vi "WriteConfiguration_Widget.vi"(7 "PythonConverter_GUI in":refnum<class "PythonConverter_GUI.lvclass">, 8 "error in":errorcluster, 11 "Control in":refnum<class "Control.lvclass">) -> (0 "error out":errorcluster, 3 "Control out":refnum<class "Control.lvclass">, 5 "PythonConverter_GUI out":refnum<class "PythonConverter_GUI.lvclass">)   [LabVIEW 2014, in "PythonConverter_GUI.lvclass"]
uses:
  PythonConverter_GUI.lvclass
  VI Interpreter/Classes/Control/Control.lvclass
  VI Interpreter/Classes/Control/Control.lvclass/Control.ctl
  PythonConverter_GUI.lvclass/PythonConverter_GUI.ctl
  PythonConfiguration/PythonConfiguration.lvclass/PythonConfiguration.ctl
  VI Interpreter/Classes/Boolean/Boolean.lvclass/Boolean.ctl
  VI Interpreter/Classes/Digital/Digital.lvclass/Digital.ctl
  VI Interpreter/Classes/Text/Text.lvclass/Text.ctl
  VI Interpreter/Classes/GraphChart/GraphChart.lvclass/GraphChart.ctl
  VI Interpreter/Classes/GraphScale/GraphScale.lvclass/GraphScale.ctl
  VI Interpreter/Classes/WaveformGraph/WaveformGraph.lvclass/WaveformGraph.ctl
  VI Interpreter/Classes/Knob/Knob.lvclass/Knob.ctl
  VI Interpreter/Classes/RotaryColorScale/RotaryColorScale.lvclass/RotaryColorScale.ctl
  VI Interpreter/Classes/NumericWithScale/NumericWithScale.lvclass/NumericWithScale.ctl
  VI Interpreter/Classes/Scale/Scale.lvclass/Scale.ctl
  VI Interpreter/Classes/String/String.lvclass/String.ctl
  VI Interpreter/Classes/IOName/IOName.lvclass/IOName.ctl
  VI Interpreter/Classes/Path/Path.lvclass/Path.ctl
  <vilib>/Utility/miscctls.llb/LVPositionTypeDef.ctl
  VI Interpreter/Classes/GObject/GObject.lvclass/GObject.ctl
  VI Interpreter/Classes/Combobox/Combobox.lvclass/Combobox.ctl
  VI Interpreter/Classes/Ring/Ring.lvclass/Ring.ctl
  VI Interpreter/Classes/Array/Array.lvclass/Array.ctl
  VI Interpreter/Classes/Cluster/Cluster.lvclass/Cluster.ctl
  VI Interpreter/Classes/NamedNumeric/NamedNumeric.lvclass/NamedNumeric.ctl
  VI Interpreter/Classes/Slide/Slide.lvclass/Slide.ctl
  VI Interpreter/Classes/Decoration/Decoration.lvclass/Decoration.ctl
  VI Interpreter/Classes/PageSelector/PageSelector.lvclass/PageSelector.ctl
  VI Interpreter/Classes/Page/Page.lvclass/Page.ctl
  VI Interpreter/Classes/Tab/Tab.lvclass/Tab.ctl
  VI Interpreter/Classes/Boolean/Boolean.lvclass
  VI Interpreter/Classes/Knob/Knob.lvclass
  VI Interpreter/Classes/Path/Path.lvclass
  VI Interpreter/Classes/Tab/Tab.lvclass
  PythonConfiguration/PythonConfiguration.lvclass
  VI Interpreter/Classes/GObject/GObject.lvclass
  VI Interpreter/Classes/Decoration/Decoration.lvclass
  VI Interpreter/Classes/Text/Text.lvclass
  VI Interpreter/Classes/PageSelector/PageSelector.lvclass
  VI Interpreter/Classes/Page/Page.lvclass
  VI Interpreter/Classes/RotaryColorScale/RotaryColorScale.lvclass
  VI Interpreter/Classes/Slide/Slide.lvclass
  VI Interpreter/Classes/Scale/Scale.lvclass
  VI Interpreter/Classes/String/String.lvclass
  VI Interpreter/Classes/Combobox/Combobox.lvclass
  VI Interpreter/Classes/Ring/Ring.lvclass
  VI Interpreter/Classes/NamedNumeric/NamedNumeric.lvclass
  VI Interpreter/Classes/Enum/Enum.lvclass
  VI Interpreter/Classes/NumericWithScale/NumericWithScale.lvclass
  VI Interpreter/Classes/Digital/Digital.lvclass
  VI Interpreter/Classes/Array/Array.lvclass
  VI Interpreter/Classes/Cluster/Cluster.lvclass
  VI Interpreter/Classes/VisaResourceName/VisaResourceName.lvclass
  VI Interpreter/Classes/IOName/IOName.lvclass
  VI Interpreter/Classes/GraphChart/GraphChart.lvclass
  VI Interpreter/Classes/GraphScale/GraphScale.lvclass
  VI Interpreter/Classes/WaveformGraph/WaveformGraph.lvclass
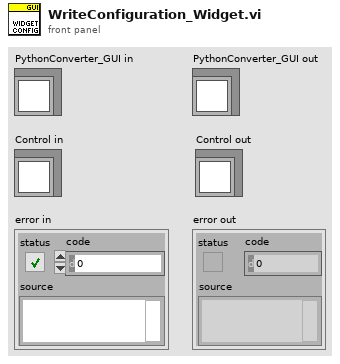
[diagram p1: front panel]
types:
  T1 = typedef "PythonConverter_GUI.lvclass/ConstructorInfo.ctl" = cluster{"Style ID":u32, "python class":string, "python module":string, "python module name":string, "check datatype":bool, "get image":bool}
  T2 = typedef "LVBoundsTypeDef.ctl" = cluster{"Width":u32, "Height":u32}
  T3 = typedef "LVPositionTypeDef.ctl" = cluster{"Left":i32, "Top":i32}
  T4 = typedef "PythonConfiguration.lvclass/ItemTD.ctl" = cluster{"Key":string, "Value":string}
  T5 = typedef "LVFontTypeDef.ctl" = cluster{"Font Name":string, "Size":u16, "Bold":bool, "Italic":bool, "Underline":bool, "Strikeout":bool, "Color":u32}
  T6 = cluster{"Foreground Color":u32, "Background Color":u32}
  T7 = typedef "LVScalePositionTypeDef.ctl" = cluster{"Start":dbl, "Range":dbl}
  T8 = typedef "LVRangeTypeDef.ctl" = cluster{"Minimum":dbl, "Maximum":dbl, "Increment":dbl, "Minor Increment":dbl, "Start":dbl}
  T9 = typedef "LVRectTypeDef.ctl" = cluster{"Left":i16, "Top":i16, "Right":i16, "Bottom":i16}
  T10 = typedef "LVBrowseOptionsTypeDef.ctl" = cluster{"Prompt":string, "Match Pattern":string, "Mode":enum32{"existing file", "new file", "new or existing file", "existing dir", "new dir", "new or existing dir", "existing file (use LLBs)", "new file (use LLBs)", "new or existing file (use LLBs)", "new or existing file or directory (use LLBs)", "existing dir (use LLBs)", "new dir (use LLBs)", "new or existing dir (use LLBs)", "existing file or dir", "new file or dir", "new or existing file or dir", "existing file or dir (use LLBs)", "new file or dir (use LLBs)"}, "Start Path":path, "Pattern Label":string, "Button Text":string}
  T11 = enum32{"existing file", "new file", "new or existing file", "existing dir", "new dir", "new or existing dir", "existing file (use LLBs)", "new file (use LLBs)", "new or existing file (use LLBs)", "new or existing file or directory (use LLBs)", "existing dir (use LLBs)", "new dir (use LLBs)", "new or existing dir (use LLBs)", "existing file or dir", "new file or dir", "new or existing file or dir", "existing file or dir (use LLBs)", "new file or dir (use LLBs)"}
  T12 = typedef "LVComboBoxStrsAndValuesArrayTypeDef.ctl" = cluster{"String":string, "Value":string}[]
  T13 = typedef "LVForegroundBackgroundColorsTypeDef.ctl" = cluster{"Foreground Color":u32, "Background Color":u32}
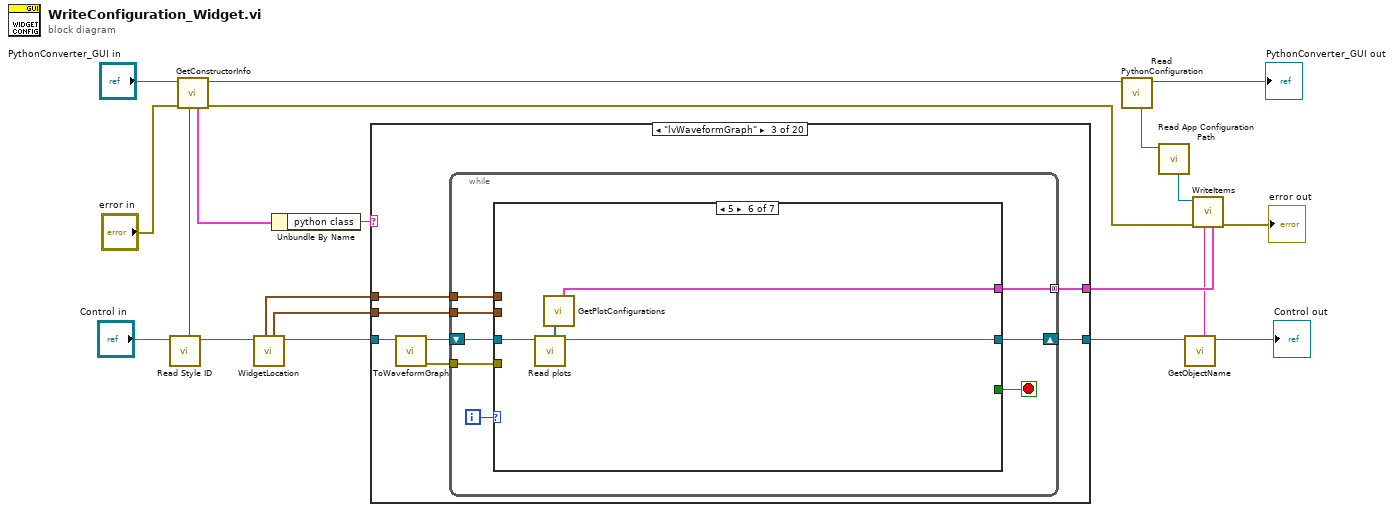
[diagram p0: block diagram]
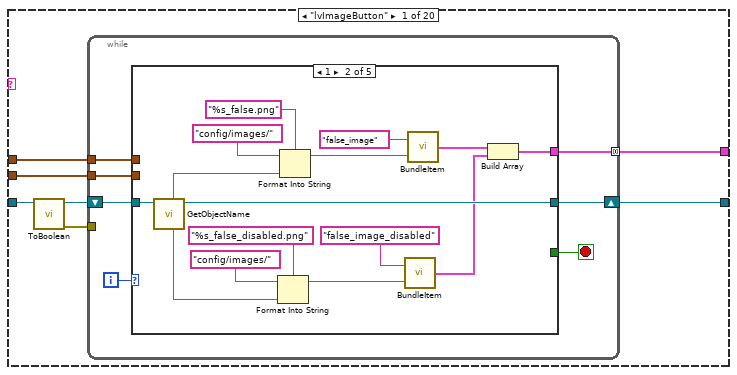
[diagram p2: hidden frame]
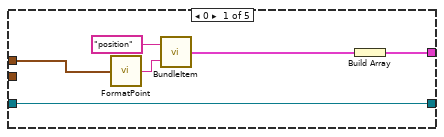
[diagram p3: hidden frame]
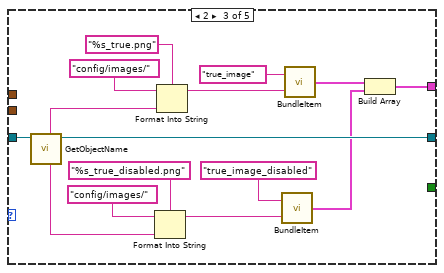
[diagram p4: hidden frame]
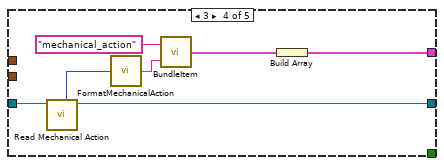
[diagram p5: hidden frame]
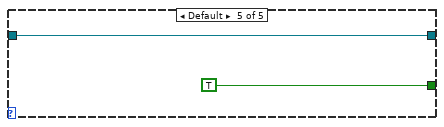
[diagram p6: hidden frame]
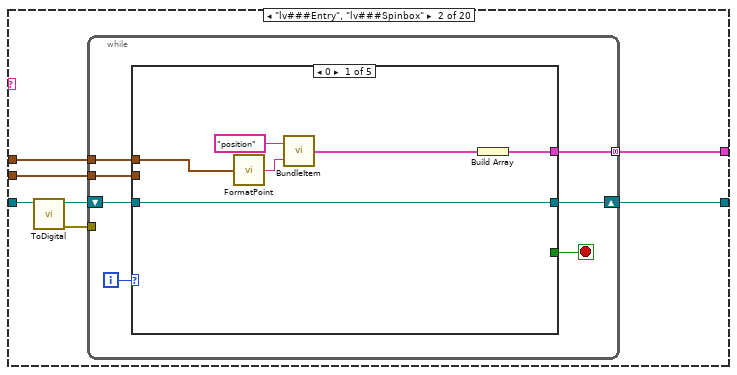
[diagram p7: hidden frame]
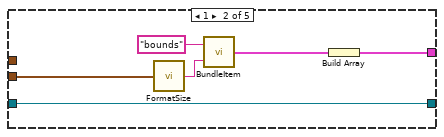
[diagram p8: hidden frame]
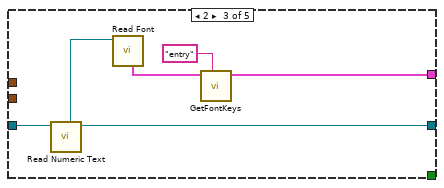
[diagram p9: hidden frame]
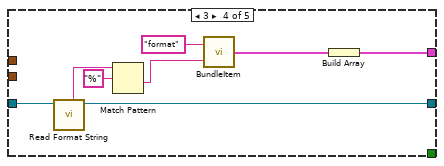
[diagram p10: hidden frame]
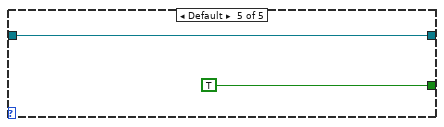
[diagram p11: hidden frame]
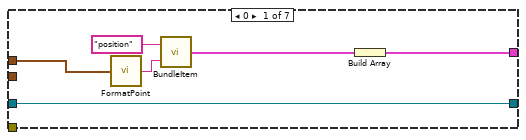
[diagram p12: hidden frame]
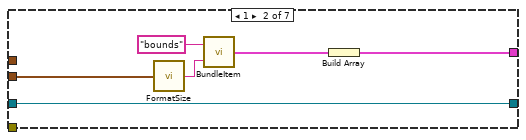
[diagram p13: hidden frame]
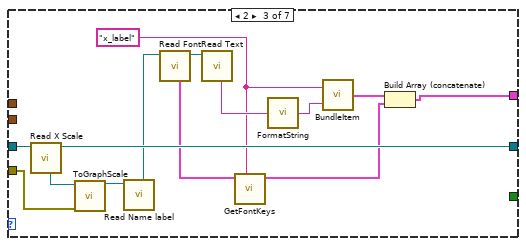
[diagram p14: hidden frame]
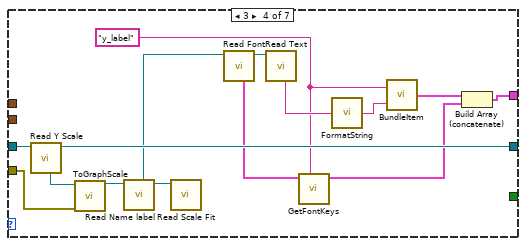
[diagram p15: hidden frame]
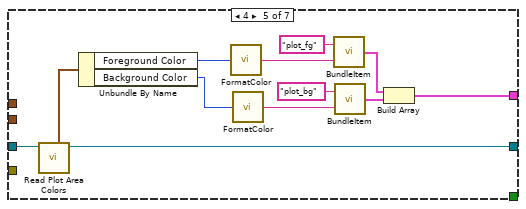
[diagram p16: hidden frame]
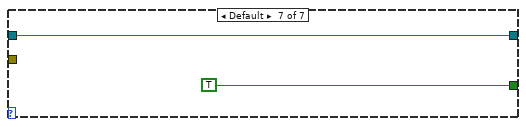
[diagram p17: hidden frame]
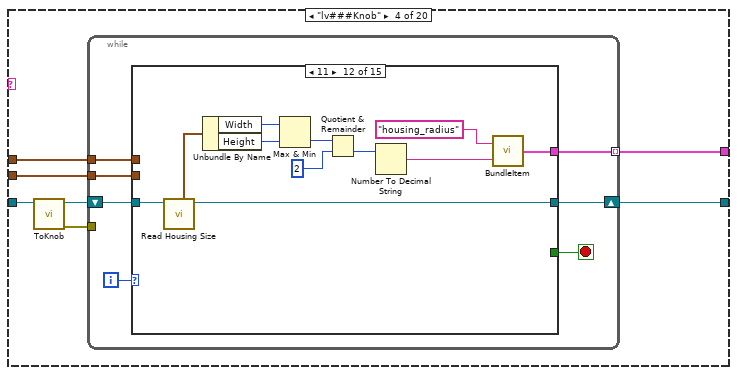
[diagram p18: hidden frame]
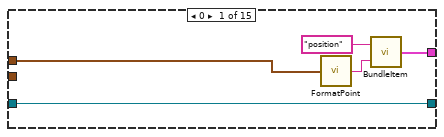
[diagram p19: hidden frame]
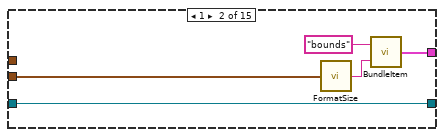
[diagram p20: hidden frame]
diagram:
  n1 = call "Read Style ID.vi"("Control in"="Control in") -> ("Control out"=w4:refnum<class "Control.lvclass">, "Style ID"=w20:u32)  [unwired: 7 in]
  n2 = call "GetConstructorInfo.vi"("Style ID"=w20, "error in"="error in", "PythonConverter_GUI in"="PythonConverter_GUI in") -> ("error out"=w5:errorcluster, "PythonConverter_GUI out"=w6:refnum<class "PythonConverter_GUI.lvclass">, "Constructor Info"=w7:T1)  [unwired: 5 in, 1 out]
  n3 = call-dynamic "WidgetLocation.vi"("Control in"=w4) -> ("Control out"=w3:refnum<class "Control.lvclass">, "Bounds"=w1:T2, "Location"=w2:T3)  [unwired: 5 in, 1 out]
  n4 = Unbundle By Name(w7) -> ("python class"=w18:string)
  n5 = case shown="\"lvWaveformGraph\"" w18 {
    tunnel: w3 -> [w24 w81 w123 w197 w326 w395 w435 w524 w580 w631 w700 w739 w774 w927 w1021 w1077 w1121 w1198 w1252 w1289]
    tunnel: [w26 w83 w125 w199 w328 w397 w437 w529 w585 w636 w705 w744 w776 w929 w1023 w1079 w1123 w1200 w1254 w1287] -> w12
    tunnel: [w27 w84 w126 w200 w329 w398 w438 w530 w586 w637 w706 w745 w777 w930 w1024 w1080 w1124 w1201 w1255 w1288] -> w14
    tunnel: w2 -> [w25 w82 w124 w198 w327 w396 w436 w528 w584 w635 w704 w743 w775 w928 w1022 w1078 w1122 w1199 w1253 w1286]
    tunnel: w1 -> [w21 w78 w120 w194 w323 w392 w432 w525 w581 w632 w701 w740 w771 w924 w1018 w1074 w1118 w1195 w1249 w1285]
    frame "lvImageButton" {
      n6 = call "ToBoolean.vi"("Generic in"=w24) -> ("error out"=w22:errorcluster, "Boolean out"=w23:refnum<class "Boolean.lvclass">)  [unwired: 9 in]
      n7 = while {
        shift-right: [w32] -> w26
        shift-left: w23 -> [w33]
        tunnel: [w31] -> w27 mode=concatenating
        tunnel: w25 -> [w29]
        tunnel: w22 -> [_]
        tunnel: w21 -> [w28]
        i -> [w34]
        stop <- w30 stop-if-true
        n8 = case shown="1" w34 {
          tunnel: w33 -> [w36 w52 w66 w72 w77]
          tunnel: [w36 w51 w65 w71 w77] -> w32
          tunnel: [w35 w47 w61 w69 _] -> w31
          tunnel: [_ _ _ _ TRUE] -> w30
          tunnel: w29 -> [w37 _ _ _ _]
          tunnel: w28 -> [_ _ _ _ _]
          frame 0 {
            n9 = call "FormatPoint.vi"("point"=w37) -> ("value"=w39:string)
            n10 = call "BundleItem.vi"("Value"=w39, "Key"="position") -> ("Item"=w38:T4)
            n11 = Build Array(w38) -> (w35:T4[])
          }
          frame 1 {
            n12 = call-dynamic "GetObjectName.vi"("GObject in"=w52) -> ("GObject out"=w51:refnum<class "Boolean.lvclass">, "Name"=w43:string)  [unwired: 6 in, 1 out]
            n13 = Format Into String(format string="%s_false_disabled.png", initial string="config/images/", w43) -> (resulting string=w45:string)  [unwired: 1 in, 1 out]
            n14 = Format Into String(format string="%s_false.png", initial string="config/images/", w43) -> (resulting string=w50:string)  [unwired: 1 in, 1 out]
            n15 = call "BundleItem.vi"("Value"=w45, "Key"="false_image_disabled") -> ("Item"=w42:T4)
            n16 = call "BundleItem.vi"("Value"=w50, "Key"="false_image") -> ("Item"=w53:T4)
            n17 = Build Array(w53, w42) -> (w47:T4[])
          }
          frame 2 {
            n18 = call-dynamic "GetObjectName.vi"("GObject in"=w66) -> ("GObject out"=w65:refnum<class "Boolean.lvclass">, "Name"=w57:string)  [unwired: 6 in, 1 out]
            n19 = Format Into String(format string="%s_true_disabled.png", initial string="config/images/", w57) -> (resulting string=w59:string)  [unwired: 1 in, 1 out]
            n20 = Format Into String(format string="%s_true.png", initial string="config/images/", w57) -> (resulting string=w64:string)  [unwired: 1 in, 1 out]
            n21 = call "BundleItem.vi"("Value"=w59, "Key"="true_image_disabled") -> ("Item"=w56:T4)
            n22 = call "BundleItem.vi"("Value"=w64, "Key"="true_image") -> ("Item"=w67:T4)
            n23 = Build Array(w67, w56) -> (w61:T4[])
          }
          frame 3 {
            n24 = call "Read Mechanical Action.vi"("Boolean in"=w72) -> ("Boolean out"=w71:refnum<class "Boolean.lvclass">, "Mechanical Action"=w70:u32)  [unwired: 7 in]
            n25 = call "FormatMechanicalAction.vi"("mechanical action"=w70) -> ("value"=w74:string)
            n26 = call "BundleItem.vi"("Value"=w74, "Key"="mechanical_action") -> ("Item"=w73:T4)
            n27 = Build Array(w73) -> (w69:T4[])
          }
          frame Default {
          }
        }
      }
    }
    frame "lv###Entry", "lv###Spinbox" {
      n28 = call "ToDigital.vi"("Generic in"=w81) -> ("error out"=w79:errorcluster, "Control out"=w80:refnum<class "Digital.lvclass">)  [unwired: 9 in]
      n29 = while {
        shift-right: [w89] -> w83
        shift-left: w80 -> [w90]
        tunnel: [w88] -> w84 mode=concatenating
        tunnel: w82 -> [w86]
        tunnel: w79 -> [_]
        tunnel: w78 -> [w85]
        i -> [w91]
        stop <- w87 stop-if-true
        n30 = case shown="0" w91 {
          tunnel: w90 -> [w93 w98 w109 w114 w119]
          tunnel: [w93 w98 w107 w113 w119] -> w89
          tunnel: [w92 w99 w106 w115 _] -> w88
          tunnel: [_ _ _ _ TRUE] -> w87
          tunnel: w86 -> [w94 _ _ _ _]
          tunnel: w85 -> [_ w101 _ _ _]
          frame 0 {
            n31 = call "FormatPoint.vi"("point"=w94) -> ("value"=w96:string)
            n32 = call "BundleItem.vi"("Value"=w96, "Key"="position") -> ("Item"=w95:T4)
            n33 = Build Array(w95) -> (w92:T4[])
          }
          frame 1 {
            n34 = call "FormatSize.vi"("size"=w101) -> ("value"=w102:string)
            n35 = call "BundleItem.vi"("Value"=w102, "Key"="bounds") -> ("Item"=w100:T4)
            n36 = Build Array(w100) -> (w99:T4[])
          }
          frame 2 {
            n37 = call "Read Numeric Text.vi"("Digital in"=w109) -> ("Digital out"=w107:refnum<class "Digital.lvclass">, "NumericText"=w108:refnum<class "NumericText.lvclass">)  [unwired: 7 in]
            n38 = call "Read Font.vi"("Text in"=w108) -> ("Font"=w105:T5)  [unwired: 7 in, 1 out]
            n39 = call "GetFontKeys.vi"("name"="entry", "Font"=w105) -> ("font items"=w106:T4[])  [unwired: 7 in]
          }
          frame 3 {
            n40 = call "Read Format String.vi"("NumericText in"=w114) -> ("NumericText out"=w113:refnum<class "Digital.lvclass">, "Format String"=w112:string)  [unwired: 7 in]
            n41 = Match Pattern(string=w112, regular expression="%") -> (after substring=w111:string)  [unwired: 1 in, 3 out]
            n42 = call "BundleItem.vi"("Value"=w111, "Key"="format") -> ("Item"=w116:T4)
            n43 = Build Array(w116) -> (w115:T4[])
          }
          frame Default {
          }
        }
      }
    }
    frame "lvWaveformGraph" {
      n44 = call "ToWaveformGraph.vi"("Generic in"=w123) -> ("error out"=w121:errorcluster, "WFGraph out"=w122:refnum<class "WaveformGraph.lvclass">)  [unwired: 9 in]
      n45 = while {
        shift-right: [w132] -> w125
        shift-left: w122 -> [w133]
        tunnel: [w131] -> w126 mode=concatenating
        tunnel: w124 -> [w129]
        tunnel: w121 -> [w127]
        tunnel: w120 -> [w128]
        i -> [w134]
        stop <- w130 stop-if-true
        n46 = case shown="5" w134 {
          tunnel: w133 -> [w136 w141 w160 w175 w187 w191 w193]
          tunnel: [w136 w141 w156 w171 w183 w190 w193] -> w132
          tunnel: [w135 w142 w153 w168 w178 w188 _] -> w131
          tunnel: [_ _ _ _ _ _ TRUE] -> w130
          tunnel: w129 -> [w137 _ _ _ _ _ _]
          tunnel: w128 -> [_ w144 _ _ _ _ _]
          tunnel: w127 -> [_ _ w158 w173 _ _ _]
          frame 0 {
            n47 = call "FormatPoint.vi"("point"=w137) -> ("value"=w139:string)
            n48 = call "BundleItem.vi"("Value"=w139, "Key"="position") -> ("Item"=w138:T4)
            n49 = Build Array(w138) -> (w135:T4[])
          }
          frame 1 {
            n50 = call "FormatSize.vi"("size"=w144) -> ("value"=w145:string)
            n51 = call "BundleItem.vi"("Value"=w145, "Key"="bounds") -> ("Item"=w143:T4)
            n52 = Build Array(w143) -> (w142:T4[])
          }
          frame 2 {
            w148 = "x_label" ("Key")
            n53 = call "Read X Scale.vi"("GraphChart in"=w160) -> ("GraphChart out"=w156:refnum<class "WaveformGraph.lvclass">, "X scale"=w159:refnum<class "GraphScale.lvclass">)  [unwired: 7 in]
            n54 = call "ToGraphScale.vi"("error in"=w158, "Generic in"=w159) -> ("GraphScale out"=w157:refnum<class "GraphScale.lvclass">)  [unwired: 8 in, 1 out]
            n55 = call "Read Name label.vi"("GraphScale in"=w157) -> ("Name label"=w150:refnum<class "Text.lvclass">)  [unwired: 7 in, 1 out]
            n56 = call "Read Font.vi"("Text in"=w150) -> ("Text out"=w151:refnum<class "Text.lvclass">, "Font"=w149:T5)  [unwired: 7 in]
            n57 = call "Read Text.vi"("Text in"=w151) -> ("Text"=w155:string)  [unwired: 7 in, 1 out]
            n58 = call "GetFontKeys.vi"("name"=w148, "Font"=w149) -> ("font items"=w147:T4[])  [unwired: 7 in]
            n59 = call "FormatString.vi"("String"=w155) -> ("value"=w154:string)  [unwired: 1 in]
            n60 = call "BundleItem.vi"("Value"=w154, "Key"=w148) -> ("Item"=w152:T4)
            n61 = Build Array (concatenate)(w152, w147) -> (w153:T4[])
          }
          frame 3 {
            w163 = "y_label" ("Key")
            n62 = call "Read Y Scale.vi"("GraphChart in"=w175) -> ("GraphChart out"=w171:refnum<class "WaveformGraph.lvclass">, "Y scale"=w174:refnum<class "GraphScale.lvclass">)  [unwired: 7 in]
            n63 = call "ToGraphScale.vi"("error in"=w173, "Generic in"=w174) -> ("GraphScale out"=w172:refnum<class "GraphScale.lvclass">)  [unwired: 8 in, 1 out]
            n64 = call "Read Name label.vi"("GraphScale in"=w172) -> ("GraphScale out"=w161:refnum<class "GraphScale.lvclass">, "Name label"=w165:refnum<class "Text.lvclass">)  [unwired: 7 in]
            n65 = call "Read Scale Fit.vi"("GraphScale in"=w161) -> ()  [unwired: 7 in, 2 out]
            n66 = call "Read Font.vi"("Text in"=w165) -> ("Text out"=w166:refnum<class "Text.lvclass">, "Font"=w164:T5)  [unwired: 7 in]
            n67 = call "Read Text.vi"("Text in"=w166) -> ("Text"=w170:string)  [unwired: 7 in, 1 out]
            n68 = call "GetFontKeys.vi"("name"=w163, "Font"=w164) -> ("font items"=w162:T4[])  [unwired: 7 in]
            n69 = call "FormatString.vi"("String"=w170) -> ("value"=w169:string)  [unwired: 1 in]
            n70 = call "BundleItem.vi"("Value"=w169, "Key"=w163) -> ("Item"=w167:T4)
            n71 = Build Array (concatenate)(w167, w162) -> (w168:T4[])
          }
          frame 4 {
            n72 = call "Read Plot Area Colors.vi"("GraphChart in"=w187) -> ("GraphChart out"=w183:refnum<class "WaveformGraph.lvclass">, "Plot Area Colors"=w186:T6)  [unwired: 7 in]
            n73 = Unbundle By Name(w186) -> ("Foreground Color"=w185:u32, "Background Color"=w184:u32)
            n74 = call "FormatColor.vi"("color"=w185) -> ("value"=w182:string)
            n75 = call "FormatColor.vi"("color"=w184) -> ("value"=w181:string)
            n76 = call "BundleItem.vi"("Value"=w182, "Key"="plot_fg") -> ("Item"=w180:T4)
            n77 = call "BundleItem.vi"("Value"=w181, "Key"="plot_bg") -> ("Item"=w179:T4)
            n78 = Build Array(w180, w179) -> (w178:T4[])
          }
          frame 5 {
            n79 = call "Read plots.vi"("WaveformChart in"=w191) -> ("WaveformChart out"=w190:refnum<class "WaveformGraph.lvclass">, "plots"=w189:refnum<class "Plot.lvclass">[])  [unwired: 7 in]
            n80 = call "GetPlotConfigurations.vi"("plots"=w189) -> ("plots cfg"=w188:T4[])  [unwired: 8 in]
          }
          frame Default {
          }
        }
      }
    }
    frame "lv###Knob" {
      n81 = call "ToKnob.vi"("Generic"=w197) -> ("error out"=w195:errorcluster, "Knob out"=w196:refnum<class "Knob.lvclass">)  [unwired: 9 in]
      n82 = while {
        shift-right: [w205] -> w199
        shift-left: w196 -> [w206]
        tunnel: [w204] -> w200 mode=indexing
        tunnel: w198 -> [w202]
        tunnel: w195 -> [_]
        tunnel: w194 -> [w201]
        i -> [w207]
        stop <- w203 stop-if-true
        n83 = case shown="11" w207 {
          tunnel: w206 -> [w208 w214 w228 w241 w249 w257 w265 w273 w281 w287 w290 w302 w309 w317 w322]
          tunnel: [w208 w214 w227 w240 w248 w256 w264 w272 w278 w284 w289 w301 w308 w316 w322] -> w205
          tunnel: [w210 w215 w229 w242 w250 w258 w266 w274 w279 w285 w292 w303 w311 w319 _] -> w204
          tunnel: [_ _ _ _ _ _ _ _ _ _ _ _ _ _ TRUE] -> w203
          tunnel: w202 -> [w209 _ _ _ _ _ _ _ _ _ _ _ _ _ _]
          tunnel: w201 -> [_ w213 _ _ _ _ _ _ _ _ _ _ _ _ _]
          frame 0 {
            n84 = call "FormatPoint.vi"("point"=w209) -> ("value"=w211:string)
            n85 = call "BundleItem.vi"("Value"=w211, "Key"="position") -> ("Item"=w210:T4)
          }
          frame 1 {
            n86 = call "FormatSize.vi"("size"=w213) -> ("value"=w216:string)
            n87 = call "BundleItem.vi"("Value"=w216, "Key"="bounds") -> ("Item"=w215:T4)
          }
          frame 2 {
            n88 = call "Read Scale.vi"("Knob in"=w228) -> ("Knob out"=w227:refnum<class "Knob.lvclass">, "Scale"=w226:refnum<class "Scale.lvclass">)  [unwired: 7 in]
            n89 = call "ToRotaryScale.vi"("Generic in"=w226) -> ("RotaryColorScale out"=w225:refnum<class "RotaryColorScale.lvclass">)  [unwired: 9 in, 1 out]
            n90 = call "Read Scale Position.vi"("RotaryColorScale in"=w225) -> ("Scale Position"=w224:T7)  [unwired: 7 in, 1 out]
            n91 = Unbundle By Name(w224) -> ("Start"=w223:dbl)
            n92 = Divide(x=w223, y=3.141592653589793) -> (x/y=w221:dbl)
            n93 = Multiply(x=180.0, y=w221) -> (x*y=w219:dbl)
            n94 = call "FormatDouble.vi"("double"=w219) -> ("value"=w218:string)
            n95 = call "BundleItem.vi"("Value"=w218, "Key"="start_angle") -> ("Item"=w229:T4)
          }
          frame 3 {
            n96 = call "Read Scale.vi"("Knob in"=w241) -> ("Knob out"=w240:refnum<class "Knob.lvclass">, "Scale"=w239:refnum<class "Scale.lvclass">)  [unwired: 7 in]
            n97 = call "ToRotaryScale.vi"("Generic in"=w239) -> ("RotaryColorScale out"=w238:refnum<class "RotaryColorScale.lvclass">)  [unwired: 9 in, 1 out]
            n98 = call "Read Scale Position.vi"("RotaryColorScale in"=w238) -> ("Scale Position"=w237:T7)  [unwired: 7 in, 1 out]
            n99 = Unbundle By Name(w237) -> ("Range"=w233:dbl)
            n100 = Divide(x=w233, y=3.141592653589793) -> (x/y=w235:dbl)
            n101 = Multiply(x=180.0, y=w235) -> (x*y=w232:dbl)
            n102 = call "FormatDouble.vi"("double"=w232) -> ("value"=w231:string)
            n103 = call "BundleItem.vi"("Value"=w231, "Key"="span") -> ("Item"=w242:T4)
          }
          frame 4 {
            n104 = call-dynamic "GetObjectName.vi"("GObject in"=w249) -> ("GObject out"=w248:refnum<class "Knob.lvclass">, "Name"=w247:string)  [unwired: 6 in, 1 out]
            n105 = Format Into String(format string="%s_housing.png", initial string="config/images/", w247) -> (resulting string=w246:string)  [unwired: 1 in, 1 out]
            n106 = call "BundleItem.vi"("Value"=w246, "Key"="housing_image") -> ("Item"=w250:T4)
          }
          frame 5 {
            n107 = call-dynamic "GetObjectName.vi"("GObject in"=w257) -> ("GObject out"=w256:refnum<class "Knob.lvclass">, "Name"=w255:string)  [unwired: 6 in, 1 out]
            n108 = Format Into String(format string="%s_housing_disabled.png", initial string="config/images/", w255) -> (resulting string=w254:string)  [unwired: 1 in, 1 out]
            n109 = call "BundleItem.vi"("Value"=w254, "Key"="housing_image_disabled") -> ("Item"=w258:T4)
          }
          frame 6 {
            n110 = call-dynamic "GetObjectName.vi"("GObject in"=w265) -> ("GObject out"=w264:refnum<class "Knob.lvclass">, "Name"=w263:string)  [unwired: 6 in, 1 out]
            n111 = Format Into String(format string="%s_marker.png", initial string="config/images/", w263) -> (resulting string=w262:string)  [unwired: 1 in, 1 out]
            n112 = call "BundleItem.vi"("Value"=w262, "Key"="marker_image") -> ("Item"=w266:T4)
          }
          frame 7 {
            n113 = call-dynamic "GetObjectName.vi"("GObject in"=w273) -> ("GObject out"=w272:refnum<class "Knob.lvclass">, "Name"=w271:string)  [unwired: 6 in, 1 out]
            n114 = Format Into String(format string="%s_marker_disabled.png", initial string="config/images/", w271) -> (resulting string=w270:string)  [unwired: 1 in, 1 out]
            n115 = call "BundleItem.vi"("Value"=w270, "Key"="marker_image_disabled") -> ("Item"=w274:T4)
          }
          frame 8 {
            n116 = call "Read Snap.vi"("Knob in"=w281) -> ("Knob out"=w278:refnum<class "Knob.lvclass">, "Snap"=w276:bool)  [unwired: 7 in]
            n117 = call "FormatBoolean.vi"("boolean"=w276) -> ("value"=w277:string)
            n118 = call "BundleItem.vi"("Value"=w277, "Key"="snap") -> ("Item"=w279:T4)
          }
          frame 9 {
            n119 = call "Read Lock.vi"("Knob in"=w287) -> ("Knob out"=w284:refnum<class "Knob.lvclass">, "Lock"=w282:bool)  [unwired: 7 in]
            n120 = call "FormatBoolean.vi"("boolean"=w282) -> ("value"=w283:string)
            n121 = call "BundleItem.vi"("Value"=w283, "Key"="lock") -> ("Item"=w285:T4)
          }
          frame 10 {
            n122 = call-dynamic "WidgetCenter.vi"("Control in"=w290) -> ("Control out"=w289:refnum<class "Knob.lvclass">, "Center"=w288:T3)  [unwired: 6 in, 1 out]
            n123 = call "FormatPoint.vi"("point"=w288) -> ("value"=w291:string)
            n124 = call "BundleItem.vi"("Value"=w291, "Key"="center") -> ("Item"=w292:T4)
          }
          frame 11 {
            n125 = call "Read Housing Size.vi"("NumericWithScale in"=w302) -> ("NumericWithScale out"=w301:refnum<class "Knob.lvclass">, "Housing Size"=w300:T2)  [unwired: 7 in]
            n126 = Unbundle By Name(w300) -> ("Width"=w299:u32, "Height"=w298:u32)
            n127 = Max & Min(x=w299, y=w298) -> (min(x,y)=w296:u32)  [unwired: 1 out]
            n128 = Quotient & Remainder(x=w296, y=u32 2) -> (floor(x/y)=w295:u32)  [unwired: 1 out]
            n129 = Number To Decimal String(number=w295) -> (decimal integer string=w297:string)  [unwired: 1 in]
            n130 = call "BundleItem.vi"("Value"=w297, "Key"="housing_radius") -> ("Item"=w303:T4)
          }
          frame 12 {
            n131 = call "Read Scale.vi"("Knob in"=w309) -> ("Knob out"=w308:refnum<class "Knob.lvclass">, "Scale"=w310:refnum<class "Scale.lvclass">)  [unwired: 7 in]
            n132 = call "Read Range.vi"("Scale in"=w310) -> ("Range"=w307:T8)  [unwired: 7 in, 1 out]
            n133 = Unbundle By Name(w307) -> ("Minimum"=w305:dbl)
            n134 = call "FormatDouble.vi"("double"=w305) -> ("value"=w306:string)
            n135 = call "BundleItem.vi"("Value"=w306, "Key"="scale_min") -> ("Item"=w311:T4)
          }
          frame 13 {
            n136 = call "Read Scale.vi"("Knob in"=w317) -> ("Knob out"=w316:refnum<class "Knob.lvclass">, "Scale"=w318:refnum<class "Scale.lvclass">)  [unwired: 7 in]
            n137 = call "Read Range.vi"("Scale in"=w318) -> ("Range"=w315:T8)  [unwired: 7 in, 1 out]
            n138 = Unbundle By Name(w315) -> ("Maximum"=w313:dbl)
            n139 = call "FormatDouble.vi"("double"=w313) -> ("value"=w314:string)
            n140 = call "BundleItem.vi"("Value"=w314, "Key"="scale_max") -> ("Item"=w319:T4)
          }
          frame Default {
          }
        }
      }
    }
    frame "lvStringEntry" {
      n141 = call "ToString.vi"("String in"=w326) -> ("error out"=w324:errorcluster, "String out"=w325:refnum<class "String.lvclass">)  [unwired: 9 in]
      n142 = while {
        shift-right: [w334] -> w328
        shift-left: w325 -> [w335]
        tunnel: [w333] -> w329 mode=concatenating
        tunnel: w327 -> [w331]
        tunnel: w324 -> [_]
        tunnel: w323 -> [w330]
        i -> [w336]
        stop <- w332 stop-if-true
        n143 = case shown="7" w336 {
          tunnel: w335 -> [w338 w345 w355 w362 w369 w376 w383 w389 w391]
          tunnel: [w338 w345 w352 w359 w366 w373 w380 w388 w391] -> w334
          tunnel: [w337 w343 w349 w356 w363 w370 w377 w385 _] -> w333
          tunnel: [_ _ _ _ _ _ _ _ TRUE] -> w332
          tunnel: w331 -> [w339 _ _ _ _ _ _ _ _]
          tunnel: w330 -> [_ w344 _ _ _ _ _ _ _]
          frame 0 {
            n144 = call "FormatPoint.vi"("point"=w339) -> ("value"=w341:string)
            n145 = call "BundleItem.vi"("Value"=w341, "Key"="position") -> ("Item"=w340:T4)
            n146 = Build Array(w340) -> (w337:T4[])
          }
          frame 1 {
            n147 = call "FormatSize.vi"("size"=w344) -> ("value"=w347:string)
            n148 = call "BundleItem.vi"("Value"=w347, "Key"="bounds") -> ("Item"=w346:T4)
            n149 = Build Array(w346) -> (w343:T4[])
          }
          frame 2 {
            n150 = call "Read Vertical Scrollbar.vi"("String in"=w355) -> ("String out"=w352:refnum<class "String.lvclass">, "Vertical Scrollbar"=w350:bool)  [unwired: 7 in]
            n151 = call "FormatBoolean.vi"("boolean"=w350) -> ("value"=w351:string)
            n152 = call "BundleItem.vi"("Value"=w351, "Key"="vScroll") -> ("Item"=w353:T4)
            n153 = Build Array(w353) -> (w349:T4[])
          }
          frame 3 {
            n154 = call "Read Horizontal Scrollbar.vi"("String in"=w362) -> ("String out"=w359:refnum<class "String.lvclass">, "Horizontal Scrollbar"=w357:bool)  [unwired: 7 in]
            n155 = call "FormatBoolean.vi"("boolean"=w357) -> ("value"=w358:string)
            n156 = call "BundleItem.vi"("Value"=w358, "Key"="hScroll") -> ("Item"=w360:T4)
            n157 = Build Array(w360) -> (w356:T4[])
          }
          frame 4 {
            n158 = call "Read Single Line.vi"("String in"=w369) -> ("String out"=w366:refnum<class "String.lvclass">, "Single Line"=w364:bool)  [unwired: 7 in]
            n159 = call "FormatBoolean.vi"("boolean"=w364) -> ("value"=w365:string)
            n160 = call "BundleItem.vi"("Value"=w365, "Key"="singleLine") -> ("Item"=w367:T4)
            n161 = Build Array(w367) -> (w363:T4[])
          }
          frame 5 {
            n162 = call "Read Display Style.vi"("String in"=w376) -> ("String out"=w373:refnum<class "String.lvclass">, "Display Style"=w371:u32)  [unwired: 7 in]
            n163 = Number To Decimal String(number=w371) -> (decimal integer string=w372:string)  [unwired: 1 in]
            n164 = call "BundleItem.vi"("Value"=w372, "Key"="displayStyle") -> ("Item"=w374:T4)
            n165 = Build Array(w374) -> (w370:T4[])
          }
          frame 6 {
            n166 = call "Read Display Format Visible.vi"("String in"=w383) -> ("String out"=w380:refnum<class "String.lvclass">, "Display Format Visible"=w378:bool)  [unwired: 7 in]
            n167 = call "FormatBoolean.vi"("boolean"=w378) -> ("value"=w379:string)
            n168 = call "BundleItem.vi"("Value"=w379, "Key"="showStyle") -> ("Item"=w381:T4)
            n169 = Build Array(w381) -> (w377:T4[])
          }
          frame 7 {
            n170 = call "Read Text.vi"("String in"=w389) -> ("String out"=w388:refnum<class "String.lvclass">, "Text"=w387:refnum<class "Text.lvclass">)  [unwired: 7 in]
            n171 = call "Read Font.vi"("Text in"=w387) -> ("Font"=w384:T5)  [unwired: 7 in, 1 out]
            n172 = call "GetFontKeys.vi"("name"="entry", "Font"=w384) -> ("font items"=w385:T4[])  [unwired: 7 in]
          }
          frame Default {
          }
        }
      }
    }
    frame "lvVisaResourceName" {
      n173 = call "ToVisaResourceName.vi"("Generic"=w395) -> ("error out"=w393:errorcluster, "VisaResourceName"=w394:refnum<class "VisaResourceName.lvclass">)  [unwired: 9 in]
      n174 = while {
        shift-right: [w403] -> w397
        shift-left: w394 -> [w404]
        tunnel: [w402] -> w398 mode=concatenating
        tunnel: w396 -> [w400]
        tunnel: w393 -> [_]
        tunnel: w392 -> [w399]
        i -> [w405]
        stop <- w401 stop-if-true
        n175 = case shown="Default" w405 {
          tunnel: w404 -> [w407 w414 w419 w429 w431]
          tunnel: [w407 w414 w419 w428 w431] -> w403
          tunnel: [w406 w412 w420 w425 _] -> w402
          tunnel: [_ _ _ _ TRUE] -> w401
          tunnel: w400 -> [w408 _ _ _ _]
          tunnel: w399 -> [_ w413 _ _ _]
          frame 0 {
            n176 = call "FormatPoint.vi"("point"=w408) -> ("value"=w410:string)
            n177 = call "BundleItem.vi"("Value"=w410, "Key"="position") -> ("Item"=w409:T4)
            n178 = Build Array(w409) -> (w406:T4[])
          }
          frame 1 {
            n179 = call "FormatSize.vi"("size"=w413) -> ("value"=w416:string)
            n180 = call "BundleItem.vi"("Value"=w416, "Key"="bounds") -> ("Item"=w415:T4)
            n181 = Build Array(w415) -> (w412:T4[])
          }
          frame 2 {
            n182 = call "FormatBoolean.vi"("boolean"=TRUE) -> ("value"=w421:string)
            n183 = call "BundleItem.vi"("Value"=w421, "Key"="singleLine") -> ("Item"=w422:T4)
            n184 = Build Array(w422) -> (w420:T4[])
          }
          frame 3 {
            n185 = call "Read Text.vi"("IOName in"=w429) -> ("IOName out"=w428:refnum<class "VisaResourceName.lvclass">, "Text"=w427:refnum<class "Text.lvclass">)  [unwired: 7 in]
            n186 = call "Read Font.vi"("Text in"=w427) -> ("Font"=w424:T5)  [unwired: 7 in, 1 out]
            n187 = call "GetFontKeys.vi"("name"="entry", "Font"=w424) -> ("font items"=w425:T4[])  [unwired: 7 in]
          }
          frame Default {
          }
        }
      }
    }
    frame "lvPath" {
      n188 = call "ToPath.vi"("Path in"=w435) -> ("error out"=w433:errorcluster, "Path out"=w434:refnum<class "Path.lvclass">)  [unwired: 9 in]
      n189 = while {
        shift-right: [w443] -> w437
        shift-left: w434 -> [w444]
        tunnel: [w442] -> w438 mode=indexing
        tunnel: w436 -> [w440]
        tunnel: w433 -> [_]
        tunnel: w432 -> [w439]
        i -> [w445]
        stop <- w441 stop-if-true
        n190 = case shown="0" w445 {
          tunnel: w444 -> [w446 w452 w461 w462 w480 w484 w502 w508 w521 w523]
          tunnel: [w446 w452 w458 w463 w479 w485 w501 w507 w518 w523] -> w443
          tunnel: [w448 w453 w459 w474 w481 w496 w503 w506 w519 _] -> w442
          tunnel: [_ _ _ _ _ _ _ _ _ TRUE] -> w441
          tunnel: w440 -> [w447 _ _ w465 _ w487 _ _ _ _]
          tunnel: w439 -> [_ w451 _ _ _ _ _ _ _ _]
          frame 0 {
            n191 = call "FormatPoint.vi"("point"=w447) -> ("value"=w449:string)
            n192 = call "BundleItem.vi"("Value"=w449, "Key"="position") -> ("Item"=w448:T4)
          }
          frame 1 {
            n193 = call "FormatSize.vi"("size"=w451) -> ("value"=w454:string)
            n194 = call "BundleItem.vi"("Value"=w454, "Key"="bounds") -> ("Item"=w453:T4)
          }
          frame 2 {
            n195 = call "Read scrollbar.vi"("Path in"=w461) -> ("Path out"=w458:refnum<class "Path.lvclass">, "scrollbar"=w456:bool)  [unwired: 7 in]
            n196 = call "FormatBoolean.vi"("boolean"=w456) -> ("value"=w457:string)
            n197 = call "BundleItem.vi"("Value"=w457, "Key"="vScroll") -> ("Item"=w459:T4)
          }
          frame 3 {
            n198 = call "Read Master Bounds Rect.vi"("GObject in"=w462) -> ("GObject out"=w469:refnum<class "Path.lvclass">, "Master Bounds Rect"=w471:T9)  [unwired: 7 in]
            n199 = call "Read Total Rect.vi"("GObject in"=w469) -> ("GObject out"=w463:refnum<class "Path.lvclass">, "Total Rect"=w472:T9)  [unwired: 7 in]
            n200 = Subtract(x=w471, y=w472) -> (x-y=w473:T9)
            n201 = Unbundle By Name(w473) -> ("Left"=w466:i16, "Top"=w467:i16)
            n202 = Bundle By Name(cluster=T3 {"Left"=0, "Top"=0} ("Position"), "Left"=w466, "Top"=w467) -> (w468:T3)
            n203 = Subtract(x=w468, y=w465) -> (x-y=w464:T3)
            n204 = call "FormatPoint.vi"("point"=w464) -> ("value"=w475:string)
            n205 = call "BundleItem.vi"("Value"=w475, "Key"="textPos") -> ("Item"=w474:T4)
          }
          frame 4 {
            n206 = call "Read Master Bounds Rect.vi"("GObject in"=w480) -> ("GObject out"=w479:refnum<class "Path.lvclass">, "Master Bounds Rect"=w478:T9)  [unwired: 7 in]
            n207 = call <vilib>:"RectSize.vi"("rect"=w478) -> ("point"=w477:cluster{"x":i16, "y":i16})
            n208 = call "FormatSize.vi"("size"=w477) -> ("value"=w482:string)
            n209 = call "BundleItem.vi"("Value"=w482, "Key"="textBounds") -> ("Item"=w481:T4)
          }
          frame 5 {
            n210 = call "Read Browse Button Rect.vi"("Path in"=w484) -> ("Path out"=w491:refnum<class "Path.lvclass">, "Browse Button Rect"=w493:T9)  [unwired: 7 in]
            n211 = call "Read Total Rect.vi"("GObject in"=w491) -> ("GObject out"=w485:refnum<class "Path.lvclass">, "Total Rect"=w494:T9)  [unwired: 7 in]
            n212 = Subtract(x=w493, y=w494) -> (x-y=w495:T9)
            n213 = Unbundle By Name(w495) -> ("Left"=w488:i16, "Top"=w489:i16)
            n214 = Bundle By Name(cluster=T3 {"Left"=0, "Top"=0} ("Position"), "Left"=w488, "Top"=w489) -> (w490:T3)
            n215 = Subtract(x=w490, y=w487) -> (x-y=w486:T3)
            n216 = call "FormatPoint.vi"("point"=w486) -> ("value"=w497:string)
            n217 = call "BundleItem.vi"("Value"=w497, "Key"="browsePos") -> ("Item"=w496:T4)
          }
          frame 6 {
            n218 = call "Read Browse Button Rect.vi"("Path in"=w502) -> ("Path out"=w501:refnum<class "Path.lvclass">, "Browse Button Rect"=w500:T9)  [unwired: 7 in]
            n219 = call <vilib>:"RectSize.vi"("rect"=w500) -> ("point"=w499:cluster{"x":i16, "y":i16})
            n220 = call "FormatSize.vi"("size"=w499) -> ("value"=w504:string)
            n221 = call "BundleItem.vi"("Value"=w504, "Key"="browseBounds") -> ("Item"=w503:T4)
          }
          frame 7 {
            n222 = call-dynamic "GetObjectName.vi"("GObject in"=w508) -> ("GObject out"=w507:refnum<class "Path.lvclass">, "Name"=w512:string)  [unwired: 6 in, 1 out]
            n223 = Format Into String(format string="%s_decal.png", initial string="config/images/", w512) -> (resulting string=w511:string)  [unwired: 1 in, 1 out]
            n224 = call "BundleItem.vi"("Value"=w511, "Key"="decal") -> ("Item"=w506:T4)
          }
          frame 8 {
            n225 = call "Read Browse Options.vi"("Path in"=w521) -> ("Path out"=w518:refnum<class "Path.lvclass">, "Browse Options"=w517:T10)  [unwired: 7 in]
            n226 = Unbundle By Name(w517) -> ("Mode"=w516:T11)
            n227 = call "FormatEnum.vi"("enum"=w516) -> ("value"=w515:string)
            n228 = call "FixString.vi"("String"=w515) -> ("Fixed string"=w514:string)
            n229 = call "BundleItem.vi"("Value"=w514, "Key"="mode") -> ("Item"=w519:T4)
          }
          frame Default {
          }
        }
      }
    }
    frame "lvCombobox" {
      n230 = call "ToCombobox.vi"("Generic in"=w524) -> ("error out"=w526:errorcluster, "Combobox out"=w527:refnum<class "Combobox.lvclass">)  [unwired: 9 in]
      n231 = while {
        shift-right: [w535] -> w529
        shift-left: w527 -> [w536]
        tunnel: [w534] -> w530 mode=indexing
        tunnel: w528 -> [w532]
        tunnel: w526 -> [_]
        tunnel: w525 -> [w531]
        i -> [w537]
        stop <- w533 stop-if-true
        n232 = case shown="1" w537 {
          tunnel: w536 -> [w538 w544 w553 w559 w566 w575 w579]
          tunnel: [w538 w544 w550 w556 w563 w572 w579] -> w535
          tunnel: [w540 w545 w551 w557 w564 w573 _] -> w534
          tunnel: [_ _ _ _ _ _ TRUE] -> w533
          tunnel: w532 -> [w539 _ _ _ _ _ _]
          tunnel: w531 -> [_ w543 _ _ _ _ _]
          frame 0 {
            n233 = call "FormatPoint.vi"("point"=w539) -> ("value"=w541:string)
            n234 = call "BundleItem.vi"("Value"=w541, "Key"="position") -> ("Item"=w540:T4)
          }
          frame 1 {
            n235 = call "FormatSize.vi"("size"=w543) -> ("value"=w546:string)
            n236 = call "BundleItem.vi"("Value"=w546, "Key"="bounds") -> ("Item"=w545:T4)
          }
          frame 2 {
            n237 = call "Read Allow Undefinded Values.vi"("Combobox in"=w553) -> ("Combobox out"=w550:refnum<class "Combobox.lvclass">, "Allow Undefinded Values"=w548:bool)  [unwired: 7 in]
            n238 = call "FormatBoolean.vi"("boolean"=w548) -> ("value"=w549:string)
            n239 = call "BundleItem.vi"("Value"=w549, "Key"="allowUndefined") -> ("Item"=w551:T4)
          }
          frame 3 {
            n240 = call "Read Case sensitive.vi"("Combobox in"=w559) -> ("Combobox out"=w556:refnum<class "Combobox.lvclass">, "Case sensitive"=w554:bool)  [unwired: 7 in]
            n241 = call "FormatBoolean.vi"("boolean"=w554) -> ("value"=w555:string)
            n242 = call "BundleItem.vi"("Value"=w555, "Key"="caseSensitive") -> ("Item"=w557:T4)
          }
          frame 4 {
            n243 = call "Read Strings And Values [].vi"("Combobox in"=w566) -> ("Combobox out"=w563:refnum<class "Combobox.lvclass">, "Strings And Values []"=w561:T12)  [unwired: 7 in]
            n244 = for {
              tunnel: w561 -> [w568] mode=indexing
              tunnel: [w567] -> w560 mode=indexing
              n245 = Unbundle By Name(w568) -> ("String"=w567:string)
            }
            n246 = call "FormatStringArray.vi"("strings"=w560) -> ("value"=w562:string)  [unwired: 1 in]
            n247 = call "BundleItem.vi"("Value"=w562, "Key"="items") -> ("Item"=w564:T4)
          }
          frame 5 {
            n248 = call "Read Strings And Values [].vi"("Combobox in"=w575) -> ("Combobox out"=w572:refnum<class "Combobox.lvclass">, "Strings And Values []"=w570:T12)  [unwired: 7 in]
            n249 = for {
              tunnel: w570 -> [w577] mode=indexing
              tunnel: [w576] -> w569 mode=indexing
              n250 = Unbundle By Name(w577) -> ("Value"=w576:string)
            }
            n251 = call "FormatStringArray.vi"("strings"=w569) -> ("value"=w571:string)  [unwired: 1 in]
            n252 = call "BundleItem.vi"("Value"=w571, "Key"="values") -> ("Item"=w573:T4)
          }
          frame Default {
          }
        }
      }
    }
    frame "lvOptionMenu", "lvRing" {
      n253 = call "ToRing.vi"("Ring in"=w580) -> ("error out"=w582:errorcluster, "Ring out"=w583:refnum<class "Ring.lvclass">)  [unwired: 9 in]
      n254 = while {
        shift-right: [w591] -> w585
        shift-left: w583 -> [w592]
        tunnel: [w590] -> w586 mode=indexing
        tunnel: w584 -> [w588]
        tunnel: w582 -> [_]
        tunnel: w581 -> [w587]
        i -> [w593]
        stop <- w589 stop-if-true
        n255 = case shown="Default" w593 {
          tunnel: w592 -> [w594 w600 w609 w616 w625 w630]
          tunnel: [w594 w600 w606 w613 w622 w630] -> w591
          tunnel: [w596 w601 w607 w614 w623 _] -> w590
          tunnel: [_ _ _ _ _ TRUE] -> w589
          tunnel: w588 -> [w595 _ _ _ _ _]
          tunnel: w587 -> [_ w599 _ _ _ _]
          frame 0 {
            n256 = call "FormatPoint.vi"("point"=w595) -> ("value"=w597:string)
            n257 = call "BundleItem.vi"("Value"=w597, "Key"="position") -> ("Item"=w596:T4)
          }
          frame 1 {
            n258 = call "FormatSize.vi"("size"=w599) -> ("value"=w602:string)
            n259 = call "BundleItem.vi"("Value"=w602, "Key"="bounds") -> ("Item"=w601:T4)
          }
          frame 2 {
            n260 = call "Read Allow Undefinded Values.vi"("Ring in"=w609) -> ("Ring out"=w606:refnum<class "Ring.lvclass">, "Allow Undefinded Values"=w604:bool)  [unwired: 7 in]
            n261 = call "FormatBoolean.vi"("boolean"=w604) -> ("value"=w605:string)
            n262 = call "BundleItem.vi"("Value"=w605, "Key"="allowUndefined") -> ("Item"=w607:T4)
          }
          frame 3 {
            n263 = call "Read Strings And Values [].vi"("Ring in"=w616) -> ("Ring out"=w613:refnum<class "Ring.lvclass">, "Strings And Values []"=w611:cluster{"String":string, "Value":variant}[])  [unwired: 7 in]
            n264 = for {
              tunnel: w611 -> [w618] mode=indexing
              tunnel: [w617] -> w610 mode=indexing
              n265 = Unbundle By Name(w618) -> ("String"=w617:string)
            }
            n266 = call "FormatStringArray.vi"("strings"=w610) -> ("value"=w612:string)  [unwired: 1 in]
            n267 = call "BundleItem.vi"("Value"=w612, "Key"="items") -> ("Item"=w614:T4)
          }
          frame 4 {
            n268 = call "Read Strings And Values [].vi"("Ring in"=w625) -> ("Ring out"=w622:refnum<class "Ring.lvclass">, "Strings And Values []"=w620:cluster{"String":string, "Value":variant}[])  [unwired: 7 in]
            n269 = for {
              tunnel: w620 -> [w628] mode=indexing
              tunnel: [w626] -> w619 mode=indexing
              n270 = Unbundle By Name(w628) -> ("Value"=w627:variant)
              n271 = Variant To Flattened String(Variant=w627) -> (data string=w626:string)  [unwired: 1 out]
            }
            n272 = call "FormatStringArray.vi"("strings"=w619) -> ("value"=w621:string)  [unwired: 1 in]
            n273 = call "BundleItem.vi"("Value"=w621, "Key"="values") -> ("Item"=w623:T4)
          }
          frame Default {
          }
        }
      }
    }
    frame "lvArray" {
      n274 = call "ToArray.vi"("Generic in"=w631) -> ("error out"=w633:errorcluster, "Array out"=w634:refnum<class "Array.lvclass">)  [unwired: 9 in]
      n275 = while {
        shift-right: [w642] -> w636
        shift-left: w634 -> [w643]
        tunnel: [w641] -> w637 mode=indexing
        tunnel: w635 -> [w639]
        tunnel: w633 -> [_]
        tunnel: w632 -> [w638]
        i -> [w644]
        stop <- w640 stop-if-true
        n276 = case shown="0" w644 {
          tunnel: w643 -> [w645 w651 w658 w661 w669 w676 w681 w687 w694 w699]
          tunnel: [w645 w651 w657 w662 w668 w675 w680 w686 w693 w699] -> w642
          tunnel: [w647 w652 w659 w665 w671 w677 w683 w689 w695 _] -> w641
          tunnel: [_ _ _ _ _ _ _ _ _ TRUE] -> w640
          tunnel: w639 -> [w646 _ _ _ _ _ _ _ _ _]
          tunnel: w638 -> [_ w650 _ _ _ _ _ _ _ _]
          frame 0 {
            n277 = call "FormatPoint.vi"("point"=w646) -> ("value"=w648:string)
            n278 = call "BundleItem.vi"("Value"=w648, "Key"="position") -> ("Item"=w647:T4)
          }
          frame 1 {
            n279 = call "FormatSize.vi"("size"=w650) -> ("value"=w653:string)
            n280 = call "BundleItem.vi"("Value"=w653, "Key"="bounds") -> ("Item"=w652:T4)
          }
          frame 2 {
            n281 = call "Read Number of Dims.vi"("Array in"=w658) -> ("Array out"=w657:refnum<class "Array.lvclass">, "Number of Dims"=w655:u32)  [unwired: 7 in]
            n282 = Number To Decimal String(number=w655) -> (decimal integer string=w656:string)  [unwired: 1 in]
            n283 = call "BundleItem.vi"("Value"=w656, "Key"="nDims") -> ("Item"=w659:T4)
          }
          frame 3 {
            n284 = call "Read Number of Rows.vi"("Array in"=w661) -> ("Array out"=w662:refnum<class "Array.lvclass">, "Number of Rows"=w663:u32)  [unwired: 7 in]
            n285 = Number To Decimal String(number=w663) -> (decimal integer string=w664:string)  [unwired: 1 in]
            n286 = call "BundleItem.vi"("Value"=w664, "Key"="nRows") -> ("Item"=w665:T4)
          }
          frame 4 {
            n287 = call "Read Number of Columns.vi"("Array in"=w669) -> ("Array out"=w668:refnum<class "Array.lvclass">, "Number of Columns"=w667:u32)  [unwired: 7 in]
            n288 = Number To Decimal String(number=w667) -> (decimal integer string=w670:string)  [unwired: 1 in]
            n289 = call "BundleItem.vi"("Value"=w670, "Key"="nCols") -> ("Item"=w671:T4)
          }
          frame 5 {
            n290 = call "Read Horizontal Scrollbar Visible.vi"("Array in"=w676) -> ("Array out"=w675:refnum<class "Array.lvclass">, "Horizontal Scrollbar Visible"=w673:bool)  [unwired: 7 in]
            n291 = call "FormatBoolean.vi"("boolean"=w673) -> ("value"=w674:string)
            n292 = call "BundleItem.vi"("Value"=w674, "Key"="horScroll") -> ("Item"=w677:T4)
          }
          frame 6 {
            n293 = call "Read Vertical Scrollbar Visible.vi"("Array in"=w681) -> ("Array out"=w680:refnum<class "Array.lvclass">, "Vertical Scrollbar Visible"=w679:bool)  [unwired: 7 in]
            n294 = call "FormatBoolean.vi"("boolean"=w679) -> ("value"=w682:string)
            n295 = call "BundleItem.vi"("Value"=w682, "Key"="vertScroll") -> ("Item"=w683:T4)
          }
          frame 7 {
            n296 = call "Read Index Visible.vi"("Array in"=w687) -> ("Array out"=w686:refnum<class "Array.lvclass">, "Index Visible"=w685:bool)  [unwired: 7 in]
            n297 = call "FormatBoolean.vi"("boolean"=w685) -> ("value"=w688:string)
            n298 = call "BundleItem.vi"("Value"=w688, "Key"="indexVisible") -> ("Item"=w689:T4)
          }
          frame 8 {
            n299 = call "Read Index Rect.vi"("Array in"=w694) -> ("Array out"=w693:refnum<class "Array.lvclass">, "Index Rect"=w692:T9)  [unwired: 7 in]
            n300 = call <vilib>:"RectSize.vi"("rect"=w692) -> ("point"=w691:cluster{"x":i16, "y":i16})
            n301 = call "FormatSize.vi"("size"=w691) -> ("value"=w696:string)
            n302 = call "BundleItem.vi"("Value"=w696, "Key"="indexBounds") -> ("Item"=w695:T4)
          }
          frame Default {
          }
        }
      }
    }
    frame "lvCluster" {
      n303 = call "ToCluster.vi"("Generic"=w700) -> ("error out"=w702:errorcluster, "Cluster out"=w703:refnum<class "Cluster.lvclass">)  [unwired: 9 in]
      n304 = while {
        shift-right: [w711] -> w705
        shift-left: w703 -> [w712]
        tunnel: [w710] -> w706 mode=indexing
        tunnel: w704 -> [w708]
        tunnel: w702 -> [_]
        tunnel: w701 -> [w707]
        i -> [w713]
        stop <- w709 stop-if-true
        n305 = case shown="3" w713 {
          tunnel: w712 -> [w714 w720 w729 w736 w738]
          tunnel: [w714 w720 w724 w732 w738] -> w711
          tunnel: [w716 w721 w726 w733 _] -> w710
          tunnel: [_ _ _ _ TRUE] -> w709
          tunnel: w708 -> [w715 _ _ _ _]
          tunnel: w707 -> [_ w719 _ _ _]
          frame 0 {
            n306 = call "FormatPoint.vi"("point"=w715) -> ("value"=w717:string)
            n307 = call "BundleItem.vi"("Value"=w717, "Key"="position") -> ("Item"=w716:T4)
          }
          frame 1 {
            n308 = call "FormatSize.vi"("size"=w719) -> ("value"=w722:string)
            n309 = call "BundleItem.vi"("Value"=w722, "Key"="bounds") -> ("Item"=w721:T4)
          }
          frame 2 {
            n310 = call "Read Color.vi"("Cluster in"=w729) -> ("Cluster out"=w724:refnum<class "Cluster.lvclass">, "Color"=w725:u32)  [unwired: 7 in]
            n311 = call "FormatColor.vi"("color"=w725) -> ("value"=w727:string)
            n312 = call "BundleItem.vi"("Value"=w727, "Key"="bgColor") -> ("Item"=w726:T4)
          }
          frame 3 {
            n313 = call "Read Color.vi"("Cluster in"=w736) -> ("Cluster out"=w732:refnum<class "Cluster.lvclass">, "Color"=w731:u32)  [unwired: 7 in]
            n314 = call "DisabledColor.vi"("enabled"=w731) -> ("disabled"=w730:u32)
            n315 = call "FormatColor.vi"("color"=w730) -> ("value"=w734:string)
            n316 = call "BundleItem.vi"("Value"=w734, "Key"="bgColorDisabled") -> ("Item"=w733:T4)
          }
          frame Default {
          }
        }
      }
    }
    frame "lvEnum" {
      n317 = call "ToEnum.vi"("Ring in"=w739) -> ("error out"=w741:errorcluster, "Enum out"=w742:refnum<class "Enum.lvclass">)  [unwired: 9 in]
      n318 = while {
        shift-right: [w750] -> w744
        shift-left: w742 -> [w751]
        tunnel: [w749] -> w745 mode=indexing
        tunnel: w743 -> [w747]
        tunnel: w741 -> [_]
        tunnel: w740 -> [w746]
        i -> [w752]
        stop <- w748 stop-if-true
        n319 = case shown="0" w752 {
          tunnel: w751 -> [w753 w759 w768 w770]
          tunnel: [w753 w759 w765 w770] -> w750
          tunnel: [w755 w760 w766 _] -> w749
          tunnel: [_ _ _ TRUE] -> w748
          tunnel: w747 -> [w754 _ _ _]
          tunnel: w746 -> [_ w758 _ _]
          frame 0 {
            n320 = call "FormatPoint.vi"("point"=w754) -> ("value"=w756:string)
            n321 = call "BundleItem.vi"("Value"=w756, "Key"="position") -> ("Item"=w755:T4)
          }
          frame 1 {
            n322 = call "FormatSize.vi"("size"=w758) -> ("value"=w761:string)
            n323 = call "BundleItem.vi"("Value"=w761, "Key"="bounds") -> ("Item"=w760:T4)
          }
          frame 2 {
            n324 = call "Read Strings.vi"("NamedNumeric in"=w768) -> ("NamedNumeric out"=w765:refnum<class "Enum.lvclass">, "Strings"=w763:string[])  [unwired: 7 in]
            n325 = call "FormatStringArray.vi"("strings"=w763) -> ("value"=w764:string)  [unwired: 1 in]
            n326 = call "BundleItem.vi"("Value"=w764, "Key"="items") -> ("Item"=w766:T4)
          }
          frame Default {
          }
        }
      }
    }
    frame "lv###Dial" {
      n327 = call "ToKnob.vi"("Generic"=w774) -> ("error out"=w772:errorcluster, "Knob out"=w773:refnum<class "Knob.lvclass">)  [unwired: 9 in]
      n328 = while {
        shift-right: [w782] -> w776
        shift-left: w773 -> [w783]
        tunnel: [w781] -> w777 mode=indexing
        tunnel: w775 -> [w779]
        tunnel: w772 -> [_]
        tunnel: w771 -> [w778]
        i -> [w784]
        stop <- w780 stop-if-true
        n329 = case shown="11" w784 {
          tunnel: w783 -> [w785 w791 w805 w818 w826 w834 w841 w861 w882 w888 w891 w900 w910 w918 w923]
          tunnel: [w785 w791 w804 w817 w825 w833 w842 w862 w879 w885 w890 w899 w909 w917 w923] -> w782
          tunnel: [w787 w792 w806 w819 w827 w835 w843 w863 w880 w886 w893 w898 w908 w916 _] -> w781
          tunnel: [_ _ _ _ _ _ _ _ _ _ _ _ _ _ TRUE] -> w780
          tunnel: w779 -> [w786 _ _ _ _ _ _ _ _ _ _ _ _ _ _]
          tunnel: w778 -> [_ w790 _ _ _ _ _ _ _ _ _ _ _ _ _]
          frame 0 {
            n330 = call "FormatPoint.vi"("point"=w786) -> ("value"=w788:string)
            n331 = call "BundleItem.vi"("Value"=w788, "Key"="position") -> ("Item"=w787:T4)
          }
          frame 1 {
            n332 = call "FormatSize.vi"("size"=w790) -> ("value"=w793:string)
            n333 = call "BundleItem.vi"("Value"=w793, "Key"="bounds") -> ("Item"=w792:T4)
          }
          frame 2 {
            n334 = call "Read Scale.vi"("Knob in"=w805) -> ("Knob out"=w804:refnum<class "Knob.lvclass">, "Scale"=w803:refnum<class "Scale.lvclass">)  [unwired: 7 in]
            n335 = call "ToRotaryScale.vi"("Generic in"=w803) -> ("RotaryColorScale out"=w802:refnum<class "RotaryColorScale.lvclass">)  [unwired: 9 in, 1 out]
            n336 = call "Read Scale Position.vi"("RotaryColorScale in"=w802) -> ("Scale Position"=w801:T7)  [unwired: 7 in, 1 out]
            n337 = Unbundle By Name(w801) -> ("Start"=w800:dbl)
            n338 = Divide(x=w800, y=3.141592653589793) -> (x/y=w798:dbl)
            n339 = Multiply(x=180.0, y=w798) -> (x*y=w796:dbl)
            n340 = call "FormatDouble.vi"("double"=w796) -> ("value"=w795:string)
            n341 = call "BundleItem.vi"("Value"=w795, "Key"="start_angle") -> ("Item"=w806:T4)
          }
          frame 3 {
            n342 = call "Read Scale.vi"("Knob in"=w818) -> ("Knob out"=w817:refnum<class "Knob.lvclass">, "Scale"=w816:refnum<class "Scale.lvclass">)  [unwired: 7 in]
            n343 = call "ToRotaryScale.vi"("Generic in"=w816) -> ("RotaryColorScale out"=w815:refnum<class "RotaryColorScale.lvclass">)  [unwired: 9 in, 1 out]
            n344 = call "Read Scale Position.vi"("RotaryColorScale in"=w815) -> ("Scale Position"=w814:T7)  [unwired: 7 in, 1 out]
            n345 = Unbundle By Name(w814) -> ("Range"=w810:dbl)
            n346 = Divide(x=w810, y=3.141592653589793) -> (x/y=w812:dbl)
            n347 = Multiply(x=180.0, y=w812) -> (x*y=w809:dbl)
            n348 = call "FormatDouble.vi"("double"=w809) -> ("value"=w808:string)
            n349 = call "BundleItem.vi"("Value"=w808, "Key"="span") -> ("Item"=w819:T4)
          }
          frame 4 {
            n350 = call-dynamic "GetObjectName.vi"("GObject in"=w826) -> ("GObject out"=w825:refnum<class "Knob.lvclass">, "Name"=w824:string)  [unwired: 6 in, 1 out]
            n351 = Format Into String(format string="%s_housing.png", initial string="config/images/", w824) -> (resulting string=w823:string)  [unwired: 1 in, 1 out]
            n352 = call "BundleItem.vi"("Value"=w823, "Key"="housing_image") -> ("Item"=w827:T4)
          }
          frame 5 {
            n353 = call-dynamic "GetObjectName.vi"("GObject in"=w834) -> ("GObject out"=w833:refnum<class "Knob.lvclass">, "Name"=w832:string)  [unwired: 6 in, 1 out]
            n354 = Format Into String(format string="%s_housing_disabled.png", initial string="config/images/", w832) -> (resulting string=w831:string)  [unwired: 1 in, 1 out]
            n355 = call "BundleItem.vi"("Value"=w831, "Key"="housing_image_disabled") -> ("Item"=w835:T4)
          }
          frame 6 {
            n356 = call "CheckDial.vi"("Knob in"=w841) -> ("error out"=w837:errorcluster, "Knob out"=w840:refnum<class "Knob.lvclass">, "Knob"=w839:bool, "Size"=w838:i16)  [unwired: 5 in]
            n357 = case shown="True" w839 {
              tunnel: [w846 w855] -> w843
              tunnel: [w848 w854] -> w842
              tunnel: w840 -> [w848 w849]
              tunnel: w838 -> [w847 _]
              tunnel: w837 -> [_ _]
              frame False {
                n358 = Number To Decimal String(number=w847) -> (decimal integer string=w845:string)  [unwired: 1 in]
                n359 = call "BundleItem.vi"("Value"=w845, "Key"="dial_width") -> ("Item"=w846:T4)
              }
              frame True {
                n360 = call-dynamic "GetObjectName.vi"("GObject in"=w849) -> ("GObject out"=w854:refnum<class "Knob.lvclass">, "Name"=w853:string)  [unwired: 6 in, 1 out]
                n361 = Format Into String(format string="%s_marker.png", initial string="config/images/", w853) -> (resulting string=w852:string)  [unwired: 1 in, 1 out]
                n362 = call "BundleItem.vi"("Value"=w852, "Key"="marker_image") -> ("Item"=w855:T4)
              }
            }
          }
          frame 7 {
            n363 = call "CheckDial.vi"("Knob in"=w861) -> ("error out"=w857:errorcluster, "Knob out"=w860:refnum<class "Knob.lvclass">, "Knob"=w859:bool, "Size"=w858:i16)  [unwired: 5 in]
            n364 = case shown="True" w859 {
              tunnel: [w866 w875] -> w863
              tunnel: [w868 w874] -> w862
              tunnel: w860 -> [w868 w869]
              tunnel: w858 -> [w867 _]
              tunnel: w857 -> [_ _]
              frame False {
                n365 = Number To Decimal String(number=w867) -> (decimal integer string=w865:string)  [unwired: 1 in]
                n366 = call "BundleItem.vi"("Value"=w865, "Key"="dial_width") -> ("Item"=w866:T4)
              }
              frame True {
                n367 = call-dynamic "GetObjectName.vi"("GObject in"=w869) -> ("GObject out"=w874:refnum<class "Knob.lvclass">, "Name"=w873:string)  [unwired: 6 in, 1 out]
                n368 = Format Into String(format string="%s_marker_disabled.png", initial string="config/images/", w873) -> (resulting string=w872:string)  [unwired: 1 in, 1 out]
                n369 = call "BundleItem.vi"("Value"=w872, "Key"="marker_image_disabled") -> ("Item"=w875:T4)
              }
            }
          }
          frame 8 {
            n370 = call "Read Snap.vi"("Knob in"=w882) -> ("Knob out"=w879:refnum<class "Knob.lvclass">, "Snap"=w877:bool)  [unwired: 7 in]
            n371 = call "FormatBoolean.vi"("boolean"=w877) -> ("value"=w878:string)
            n372 = call "BundleItem.vi"("Value"=w878, "Key"="snap") -> ("Item"=w880:T4)
          }
          frame 9 {
            n373 = call "Read Lock.vi"("Knob in"=w888) -> ("Knob out"=w885:refnum<class "Knob.lvclass">, "Lock"=w883:bool)  [unwired: 7 in]
            n374 = call "FormatBoolean.vi"("boolean"=w883) -> ("value"=w884:string)
            n375 = call "BundleItem.vi"("Value"=w884, "Key"="lock") -> ("Item"=w886:T4)
          }
          frame 10 {
            n376 = call-dynamic "WidgetCenter.vi"("Control in"=w891) -> ("Control out"=w890:refnum<class "Knob.lvclass">, "Center"=w889:T3)  [unwired: 6 in, 1 out]
            n377 = call "FormatPoint.vi"("point"=w889) -> ("value"=w892:string)
            n378 = call "BundleItem.vi"("Value"=w892, "Key"="center") -> ("Item"=w893:T4)
          }
          frame 11 {
            n379 = call "Read Housing Size.vi"("NumericWithScale in"=w900) -> ("NumericWithScale out"=w899:refnum<class "Knob.lvclass">, "Housing Size"=w904:T2)  [unwired: 7 in]
            n380 = Unbundle By Name(w904) -> ("Width"=w903:u32, "Height"=w902:u32)
            n381 = Max & Min(x=w903, y=w902) -> (min(x,y)=w897:u32)  [unwired: 1 out]
            n382 = Quotient & Remainder(x=w897, y=u32 2) -> (floor(x/y)=w895:u32)  [unwired: 1 out]
            n383 = Number To Decimal String(number=w895) -> (decimal integer string=w901:string)  [unwired: 1 in]
            n384 = call "BundleItem.vi"("Value"=w901, "Key"="housing_radius") -> ("Item"=w898:T4)
          }
          frame 12 {
            n385 = call "Read Scale.vi"("Knob in"=w910) -> ("Knob out"=w909:refnum<class "Knob.lvclass">, "Scale"=w912:refnum<class "Scale.lvclass">)  [unwired: 7 in]
            n386 = call "Read Range.vi"("Scale in"=w912) -> ("Range"=w913:T8)  [unwired: 7 in, 1 out]
            n387 = Unbundle By Name(w913) -> ("Minimum"=w907:dbl)
            n388 = call "FormatDouble.vi"("double"=w907) -> ("value"=w906:string)
            n389 = call "BundleItem.vi"("Value"=w906, "Key"="scale_min") -> ("Item"=w908:T4)
          }
          frame 13 {
            n390 = call "Read Scale.vi"("Knob in"=w918) -> ("Knob out"=w917:refnum<class "Knob.lvclass">, "Scale"=w920:refnum<class "Scale.lvclass">)  [unwired: 7 in]
            n391 = call "Read Range.vi"("Scale in"=w920) -> ("Range"=w921:T8)  [unwired: 7 in, 1 out]
            n392 = Unbundle By Name(w921) -> ("Maximum"=w915:dbl)
            n393 = call "FormatDouble.vi"("double"=w915) -> ("value"=w914:string)
            n394 = call "BundleItem.vi"("Value"=w914, "Key"="scale_max") -> ("Item"=w916:T4)
          }
          frame Default {
          }
        }
      }
    }
    frame "lv###Slider" {
      n395 = call "ToSlide.vi"("Generic"=w927) -> ("error out"=w925:errorcluster, "Slide out"=w926:refnum<class "Slide.lvclass">)  [unwired: 9 in]
      n396 = while {
        shift-right: [w935] -> w929
        shift-left: w926 -> [w936]
        tunnel: [w934] -> w930 mode=indexing
        tunnel: w928 -> [w932]
        tunnel: w925 -> [_]
        tunnel: w924 -> [w931]
        i -> [w937]
        stop <- w933 stop-if-true
        n397 = case shown="9" w937 {
          tunnel: w936 -> [w938 w944 w950 w959 w968 w978 w987 w996 w1005 w1012 w1017]
          tunnel: [w938 w944 w954 w963 w972 w980 w989 w998 w1007 w1011 w1017] -> w935
          tunnel: [w940 w945 w955 w964 w973 w981 w990 w999 w1008 w1014 _] -> w934
          tunnel: [_ _ _ _ _ _ _ _ _ _ TRUE] -> w933
          tunnel: w932 -> [w939 _ _ _ _ _ _ _ _ _ _]
          tunnel: w931 -> [_ w943 _ _ _ _ _ _ _ _ _]
          frame 0 {
            n398 = call "FormatPoint.vi"("point"=w939) -> ("value"=w941:string)
            n399 = call "BundleItem.vi"("Value"=w941, "Key"="position") -> ("Item"=w940:T4)
          }
          frame 1 {
            n400 = call "FormatSize.vi"("size"=w943) -> ("value"=w946:string)
            n401 = call "BundleItem.vi"("Value"=w946, "Key"="bounds") -> ("Item"=w945:T4)
          }
          frame 2 {
            n402 = call "Read Scale.vi"("Slide in"=w950) -> ("Slide out"=w954:refnum<class "Slide.lvclass">, "Scale"=w953:refnum<class "Scale.lvclass">)  [unwired: 7 in]
            n403 = call "ToScale.vi"("Scale in"=w953) -> ("Scale out"=w952:refnum<class "Scale.lvclass">)  [unwired: 9 in, 1 out]
            n404 = call "Read Range.vi"("Scale in"=w952) -> ("Range"=w951:T8)  [unwired: 7 in, 1 out]
            n405 = Unbundle By Name(w951) -> ("Minimum"=w949:dbl)
            n406 = call "FormatDouble.vi"("double"=w949) -> ("value"=w948:string)
            n407 = call "BundleItem.vi"("Value"=w948, "Key"="scale_min") -> ("Item"=w955:T4)
          }
          frame 3 {
            n408 = call "Read Scale.vi"("Slide in"=w959) -> ("Slide out"=w963:refnum<class "Slide.lvclass">, "Scale"=w962:refnum<class "Scale.lvclass">)  [unwired: 7 in]
            n409 = call "ToScale.vi"("Scale in"=w962) -> ("Scale out"=w961:refnum<class "Scale.lvclass">)  [unwired: 9 in, 1 out]
            n410 = call "Read Range.vi"("Scale in"=w961) -> ("Range"=w960:T8)  [unwired: 7 in, 1 out]
            n411 = Unbundle By Name(w960) -> ("Maximum"=w958:dbl)
            n412 = call "FormatDouble.vi"("double"=w958) -> ("value"=w957:string)
            n413 = call "BundleItem.vi"("Value"=w957, "Key"="scale_max") -> ("Item"=w964:T4)
          }
          frame 4 {
            n414 = call "Read Scale.vi"("Slide in"=w968) -> ("Slide out"=w972:refnum<class "Slide.lvclass">, "Scale"=w971:refnum<class "Scale.lvclass">)  [unwired: 7 in]
            n415 = call "ToScale.vi"("Scale in"=w971) -> ("Scale out"=w970:refnum<class "Scale.lvclass">)  [unwired: 9 in, 1 out]
            n416 = call "Read Range.vi"("Scale in"=w970) -> ("Range"=w969:T8)  [unwired: 7 in, 1 out]
            n417 = Unbundle By Name(w969) -> ("Increment"=w967:dbl)
            n418 = call "FormatDouble.vi"("double"=w967) -> ("value"=w966:string)
            n419 = call "BundleItem.vi"("Value"=w966, "Key"="scale_inc") -> ("Item"=w973:T4)
          }
          frame 5 {
            n420 = call "Read Scale.vi"("Slide in"=w978) -> ("Slide out"=w980:refnum<class "Slide.lvclass">, "Scale"=w979:refnum<class "Scale.lvclass">)  [unwired: 7 in]
            n421 = call "ToScale.vi"("Scale in"=w979) -> ("Scale out"=w976:refnum<class "Scale.lvclass">)  [unwired: 9 in, 1 out]
            n422 = call "GetSlideScaleVisible.vi"("Scale"=w976) -> ("scale visible"=w975:bool)  [unwired: 7 in, 1 out]
            n423 = call "FormatBoolean.vi"("boolean"=w975) -> ("value"=w977:string)
            n424 = call "BundleItem.vi"("Value"=w977, "Key"="scale_visible") -> ("Item"=w981:T4)
          }
          frame 6 {
            n425 = call "Read Scale.vi"("Slide in"=w987) -> ("Slide out"=w989:refnum<class "Slide.lvclass">, "Scale"=w988:refnum<class "Scale.lvclass">)  [unwired: 7 in]
            n426 = call "ToScale.vi"("Scale in"=w988) -> ("error out"=w985:errorcluster, "Scale out"=w986:refnum<class "Scale.lvclass">)  [unwired: 9 in]
            n427 = call "GetSlideDigits.vi"("error in"=w985, "Scale"=w986) -> ("digits"=w984:i32)  [unwired: 5 in, 2 out]
            n428 = Number To Decimal String(number=w984) -> (decimal integer string=w983:string)  [unwired: 1 in]
            n429 = call "BundleItem.vi"("Value"=w983, "Key"="digits") -> ("Item"=w990:T4)
          }
          frame 7 {
            n430 = call "Read Scale.vi"("Slide in"=w996) -> ("Slide out"=w998:refnum<class "Slide.lvclass">, "Scale"=w997:refnum<class "Scale.lvclass">)  [unwired: 7 in]
            n431 = call "ToScale.vi"("Scale in"=w997) -> ("Scale out"=w995:refnum<class "Scale.lvclass">)  [unwired: 9 in, 1 out]
            n432 = call "Read Marker.vi"("Scale in"=w995) -> ("Marker"=w994:refnum<class "Text.lvclass">)  [unwired: 7 in, 1 out]
            n433 = call "Read Document Bounds.vi"("Text in"=w994) -> ("Document Bounds"=w992:T2)  [unwired: 7 in, 1 out]
            n434 = call "FormatSize.vi"("size"=w992) -> ("value"=w993:string)
            n435 = call "BundleItem.vi"("Value"=w993, "Key"="marker_bounds") -> ("Item"=w999:T4)
          }
          frame 8 {
            n436 = call "Read Scale.vi"("Slide in"=w1005) -> ("Slide out"=w1007:refnum<class "Slide.lvclass">, "Scale"=w1006:refnum<class "Scale.lvclass">)  [unwired: 7 in]
            n437 = call "ToScale.vi"("Scale in"=w1006) -> ("Scale out"=w1004:refnum<class "Scale.lvclass">)  [unwired: 9 in, 1 out]
            n438 = call "Read Marker.vi"("Scale in"=w1004) -> ("Marker"=w1003:refnum<class "Text.lvclass">)  [unwired: 7 in, 1 out]
            n439 = call "Read Text.vi"("Text in"=w1003) -> ("Text"=w1001:string)  [unwired: 7 in, 1 out]
            n440 = call "FormatString.vi"("String"=w1001) -> ("value"=w1002:string)  [unwired: 1 in]
            n441 = call "BundleItem.vi"("Value"=w1002, "Key"="marker_text") -> ("Item"=w1008:T4)
          }
          frame 9 {
            n442 = call "IsHorizontal.vi"("Slide in"=w1012) -> ("Slide out"=w1011:refnum<class "Slide.lvclass">, "horizontal"=w1010:bool)  [unwired: 7 in]
            n443 = call "FormatBoolean.vi"("boolean"=w1010) -> ("value"=w1013:string)
            n444 = call "BundleItem.vi"("Value"=w1013, "Key"="horizontal") -> ("Item"=w1014:T4)
          }
          frame Default {
          }
        }
      }
    }
    frame "lv###ProgressBar" {
      n445 = call "ToSlide.vi"("Generic"=w1021) -> ("error out"=w1019:errorcluster, "Slide out"=w1020:refnum<class "Slide.lvclass">)  [unwired: 9 in]
      n446 = while {
        shift-right: [w1029] -> w1023
        shift-left: w1020 -> [w1030]
        tunnel: [w1028] -> w1024 mode=indexing
        tunnel: w1022 -> [w1026]
        tunnel: w1019 -> [_]
        tunnel: w1018 -> [w1025]
        i -> [w1031]
        stop <- w1027 stop-if-true
        n447 = case shown="5" w1031 {
          tunnel: w1030 -> [w1032 w1038 w1044 w1053 w1062 w1068 w1073]
          tunnel: [w1032 w1038 w1048 w1057 w1061 w1067 w1073] -> w1029
          tunnel: [w1034 w1039 w1049 w1058 w1064 w1070 _] -> w1028
          tunnel: [_ _ _ _ _ _ TRUE] -> w1027
          tunnel: w1026 -> [w1033 _ _ _ _ _ _]
          tunnel: w1025 -> [_ w1037 _ _ _ _ _]
          frame 0 {
            n448 = call "FormatPoint.vi"("point"=w1033) -> ("value"=w1035:string)
            n449 = call "BundleItem.vi"("Value"=w1035, "Key"="position") -> ("Item"=w1034:T4)
          }
          frame 1 {
            n450 = call "FormatSize.vi"("size"=w1037) -> ("value"=w1040:string)
            n451 = call "BundleItem.vi"("Value"=w1040, "Key"="bounds") -> ("Item"=w1039:T4)
          }
          frame 2 {
            n452 = call "Read Scale.vi"("Slide in"=w1044) -> ("Slide out"=w1048:refnum<class "Slide.lvclass">, "Scale"=w1047:refnum<class "Scale.lvclass">)  [unwired: 7 in]
            n453 = call "ToScale.vi"("Scale in"=w1047) -> ("Scale out"=w1046:refnum<class "Scale.lvclass">)  [unwired: 9 in, 1 out]
            n454 = call "Read Range.vi"("Scale in"=w1046) -> ("Range"=w1045:T8)  [unwired: 7 in, 1 out]
            n455 = Unbundle By Name(w1045) -> ("Minimum"=w1043:dbl)
            n456 = call "FormatDouble.vi"("double"=w1043) -> ("value"=w1042:string)
            n457 = call "BundleItem.vi"("Value"=w1042, "Key"="scale_min") -> ("Item"=w1049:T4)
          }
          frame 3 {
            n458 = call "Read Scale.vi"("Slide in"=w1053) -> ("Slide out"=w1057:refnum<class "Slide.lvclass">, "Scale"=w1056:refnum<class "Scale.lvclass">)  [unwired: 7 in]
            n459 = call "ToScale.vi"("Scale in"=w1056) -> ("Scale out"=w1055:refnum<class "Scale.lvclass">)  [unwired: 9 in, 1 out]
            n460 = call "Read Range.vi"("Scale in"=w1055) -> ("Range"=w1054:T8)  [unwired: 7 in, 1 out]
            n461 = Unbundle By Name(w1054) -> ("Maximum"=w1052:dbl)
            n462 = call "FormatDouble.vi"("double"=w1052) -> ("value"=w1051:string)
            n463 = call "BundleItem.vi"("Value"=w1051, "Key"="scale_max") -> ("Item"=w1058:T4)
          }
          frame 4 {
            n464 = call "IsHorizontal.vi"("Slide in"=w1062) -> ("Slide out"=w1061:refnum<class "Slide.lvclass">, "horizontal"=w1060:bool)  [unwired: 7 in]
            n465 = call "FormatBoolean.vi"("boolean"=w1060) -> ("value"=w1063:string)
            n466 = call "BundleItem.vi"("Value"=w1063, "Key"="horizontal") -> ("Item"=w1064:T4)
          }
          frame 5 {
            n467 = call "Read Fill color.vi"("Slide in"=w1068) -> ("Slide out"=w1067:refnum<class "Slide.lvclass">, "Fill color"=w1066:u32)  [unwired: 7 in]
            n468 = call "FormatColor.vi"("color"=w1066) -> ("value"=w1069:string)
            n469 = call "BundleItem.vi"("Value"=w1069, "Key"="barColor") -> ("Item"=w1070:T4)
          }
          frame Default {
          }
        }
      }
    }
    frame "lvSystemTextButton" {
      n470 = call "ToBoolean.vi"("Generic in"=w1077) -> ("error out"=w1075:errorcluster, "Boolean out"=w1076:refnum<class "Boolean.lvclass">)  [unwired: 9 in]
      n471 = while {
        shift-right: [w1085] -> w1079
        shift-left: w1076 -> [w1086]
        tunnel: [w1084] -> w1080 mode=indexing
        tunnel: w1078 -> [w1082]
        tunnel: w1075 -> [_]
        tunnel: w1074 -> [w1081]
        i -> [w1087]
        stop <- w1083 stop-if-true
        n472 = case shown="0" w1087 {
          tunnel: w1086 -> [w1088 w1094 w1100 w1106 w1112 w1117]
          tunnel: [w1088 w1094 w1099 w1105 w1111 w1117] -> w1085
          tunnel: [w1090 w1095 w1101 w1107 w1113 _] -> w1084
          tunnel: [_ _ _ _ _ TRUE] -> w1083
          tunnel: w1082 -> [w1089 _ _ _ _ _]
          tunnel: w1081 -> [_ w1093 _ _ _ _]
          frame 0 {
            n473 = call "FormatPoint.vi"("point"=w1089) -> ("value"=w1091:string)
            n474 = call "BundleItem.vi"("Value"=w1091, "Key"="position") -> ("Item"=w1090:T4)
          }
          frame 1 {
            n475 = call "FormatSize.vi"("size"=w1093) -> ("value"=w1096:string)
            n476 = call "BundleItem.vi"("Value"=w1096, "Key"="bounds") -> ("Item"=w1095:T4)
          }
          frame 2 {
            n477 = call "Read Mechanical Action.vi"("Boolean in"=w1100) -> ("Boolean out"=w1099:refnum<class "Boolean.lvclass">, "Mechanical Action"=w1098:u32)  [unwired: 7 in]
            n478 = call "FormatMechanicalAction.vi"("mechanical action"=w1098) -> ("value"=w1102:string)
            n479 = call "BundleItem.vi"("Value"=w1102, "Key"="mechanical_action") -> ("Item"=w1101:T4)
          }
          frame 3 {
            n480 = call "Read Mulitple Strings.vi"("Boolean in"=w1106) -> ("Boolean out"=w1105:refnum<class "Boolean.lvclass">, "Mulitple Strings"=w1104:bool)  [unwired: 7 in]
            n481 = call "FormatBoolean.vi"("boolean"=w1104) -> ("value"=w1108:string)
            n482 = call "BundleItem.vi"("Value"=w1108, "Key"="multiple_strings") -> ("Item"=w1107:T4)
          }
          frame 4 {
            n483 = call "Read Strings.vi"("Boolean in"=w1112) -> ("Boolean out"=w1111:refnum<class "Boolean.lvclass">, "Strings"=w1110:string[])  [unwired: 7 in]
            n484 = call "FormatStringArray.vi"("strings"=w1110) -> ("value"=w1114:string)  [unwired: 1 in]
            n485 = call "BundleItem.vi"("Value"=w1114, "Key"="strings") -> ("Item"=w1113:T4)
          }
          frame Default {
          }
        }
      }
    }
    frame "lvCheckButton", "lvRadioButton" {
      n486 = call "ToBoolean.vi"("Generic in"=w1121) -> ("error out"=w1119:errorcluster, "Boolean out"=w1120:refnum<class "Boolean.lvclass">)  [unwired: 9 in]
      n487 = while {
        shift-right: [w1129] -> w1123
        shift-left: w1120 -> [w1130]
        tunnel: [w1128] -> w1124 mode=indexing
        tunnel: w1122 -> [w1126]
        tunnel: w1119 -> [_]
        tunnel: w1118 -> [w1125]
        i -> [w1131]
        stop <- w1127 stop-if-true
        n488 = case shown="Default" w1131 {
          tunnel: w1130 -> [w1132 w1137 w1144 w1151 w1158 w1173 w1183 w1194]
          tunnel: [w1132 w1137 w1143 w1150 w1157 w1167 w1185 w1194] -> w1129
          tunnel: [w1134 w1139 w1145 w1152 w1159 w1174 w1190 _] -> w1128
          tunnel: [_ _ _ _ _ _ _ TRUE] -> w1127
          tunnel: w1126 -> [w1133 _ _ _ _ w1162 w1179 _]
          tunnel: w1125 -> [_ w1138 _ _ _ _ _ _]
          frame 0 {
            n489 = call "FormatPoint.vi"("point"=w1133) -> ("value"=w1135:string)
            n490 = call "BundleItem.vi"("Value"=w1135, "Key"="position") -> ("Item"=w1134:T4)
          }
          frame 1 {
            n491 = call "FormatSize.vi"("size"=w1138) -> ("value"=w1140:string)
            n492 = call "BundleItem.vi"("Value"=w1140, "Key"="bounds") -> ("Item"=w1139:T4)
          }
          frame 2 {
            n493 = call "Read Mechanical Action.vi"("Boolean in"=w1144) -> ("Boolean out"=w1143:refnum<class "Boolean.lvclass">, "Mechanical Action"=w1142:u32)  [unwired: 7 in]
            n494 = call "FormatMechanicalAction.vi"("mechanical action"=w1142) -> ("value"=w1146:string)
            n495 = call "BundleItem.vi"("Value"=w1146, "Key"="mechanical_action") -> ("Item"=w1145:T4)
          }
          frame 3 {
            n496 = call "Read BoolText.vi"("Boolean in"=w1151) -> ("Boolean out"=w1150:refnum<class "Boolean.lvclass">, "BoolText"=w1149:refnum<class "Text.lvclass">)  [unwired: 7 in]
            n497 = call "Read Visible.vi"("Decoration in"=w1149) -> ("Visible"=w1148:bool)  [unwired: 7 in, 1 out]
            n498 = call "FormatBoolean.vi"("boolean"=w1148) -> ("value"=w1153:string)
            n499 = call "BundleItem.vi"("Value"=w1153, "Key"="show_boolean_text") -> ("Item"=w1152:T4)
          }
          frame 4 {
            n500 = call "Read BoolText.vi"("Boolean in"=w1158) -> ("Boolean out"=w1157:refnum<class "Boolean.lvclass">, "BoolText"=w1156:refnum<class "Text.lvclass">)  [unwired: 7 in]
            n501 = call "Read Text.vi"("Text in"=w1156) -> ("Text"=w1155:string)  [unwired: 7 in, 1 out]
            n502 = call "FormatString.vi"("String"=w1155) -> ("value"=w1160:string)  [unwired: 1 in]
            n503 = call "BundleItem.vi"("Value"=w1160, "Key"="boolean_text") -> ("Item"=w1159:T4)
          }
          frame 5 {
            n504 = call "Read Master Bounds Rect.vi"("GObject in"=w1173) -> ("GObject out"=w1168:refnum<class "Boolean.lvclass">, "Master Bounds Rect"=w1165:T9)  [unwired: 7 in]
            n505 = call "Read Total Rect.vi"("GObject in"=w1168) -> ("GObject out"=w1167:refnum<class "Boolean.lvclass">, "Total Rect"=w1164:T9)  [unwired: 7 in]
            n506 = Subtract(x=w1165, y=w1164) -> (x-y=w1163:T9)
            n507 = Unbundle By Name(w1163) -> ("Left"=w1171:i16, "Top"=w1170:i16)
            n508 = Bundle By Name(cluster=T3 {"Left"=0, "Top"=0} ("Position"), "Left"=w1171, "Top"=w1170) -> (w1169:T3)
            n509 = Subtract(x=w1169, y=w1162) -> (x-y=w1172:T3)
            n510 = call "FormatPoint.vi"("point"=w1172) -> ("value"=w1175:string)
            n511 = call "BundleItem.vi"("Value"=w1175, "Key"="button_position") -> ("Item"=w1174:T4)
          }
          frame 6 {
            n512 = call "Read BoolText.vi"("Boolean in"=w1183) -> ("Boolean out"=w1182:refnum<class "Boolean.lvclass">, "BoolText"=w1181:refnum<class "Text.lvclass">)  [unwired: 7 in]
            n513 = call "Read Position.vi"("GObject in"=w1181) -> ("Position"=w1177:T3)  [unwired: 7 in, 1 out]
            n514 = call "Read Total Rect.vi"("GObject in"=w1182) -> ("GObject out"=w1185:refnum<class "Boolean.lvclass">, "Total Rect"=w1180:T9)  [unwired: 7 in]
            n515 = Unbundle By Name(w1180) -> ("Left"=w1188:i16, "Top"=w1187:i16)
            n516 = Bundle By Name(cluster=T3 {"Left"=0, "Top"=0} ("Position"), "Left"=w1188, "Top"=w1187) -> (w1186:T3)
            n517 = Subtract(x=w1177, y=w1179) -> (x-y=w1178:T3)
            n518 = Subtract(x=w1178, y=w1186) -> (x-y=w1189:T3)
            n519 = call "FormatPoint.vi"("point"=w1189) -> ("value"=w1191:string)
            n520 = call "BundleItem.vi"("Value"=w1191, "Key"="text_position") -> ("Item"=w1190:T4)
          }
          frame Default {
          }
        }
      }
    }
    frame "lvTabControl" {
      n521 = call "ToTab.vi"("Generic in"=w1198) -> ("error out"=w1196:errorcluster, "Tab out"=w1197:refnum<class "Tab.lvclass">)  [unwired: 9 in]
      n522 = while {
        shift-right: [w1206] -> w1200
        shift-left: w1197 -> [w1207]
        tunnel: [w1205] -> w1201 mode=indexing
        tunnel: w1199 -> [w1203]
        tunnel: w1196 -> [_]
        tunnel: w1195 -> [w1202]
        i -> [w1208]
        stop <- w1204 stop-if-true
        n523 = case shown="3" w1208 {
          tunnel: w1207 -> [w1209 w1216 w1223 w1233 w1248]
          tunnel: [w1209 w1215 w1222 w1232 w1248] -> w1206
          tunnel: [w1211 w1217 w1224 w1234 _] -> w1205
          tunnel: [_ _ _ _ TRUE] -> w1204
          tunnel: w1203 -> [w1210 _ _ _ _]
          tunnel: w1202 -> [_ w1214 _ _ _]
          frame 0 {
            n524 = call "FormatPoint.vi"("point"=w1210) -> ("value"=w1212:string)
            n525 = call "BundleItem.vi"("Value"=w1212, "Key"="position") -> ("Item"=w1211:T4)
          }
          frame 1 {
            n526 = call-dynamic "GetControlSize.vi"("Control in"=w1216) -> ("Control out"=w1215:refnum<class "Tab.lvclass">)  [unwired: 7 in, 1 out]
            n527 = call "FormatSize.vi"("size"=w1214) -> ("value"=w1218:string)
            n528 = call "BundleItem.vi"("Value"=w1218, "Key"="bounds") -> ("Item"=w1217:T4)
          }
          frame 2 {
            n529 = call "Read Pages.vi"("PageSelector in"=w1223) -> ("PageSelector out"=w1222:refnum<class "Tab.lvclass">, "Pages"=w1221:refnum<class "Page.lvclass">[])  [unwired: 7 in]
            n530 = for {
              tunnel: w1221 -> [w1228] mode=indexing
              tunnel: [w1227] -> w1220 mode=indexing
              n531 = call "Read Label.vi"("Page in"=w1228) -> ("Label"=w1227:string)  [unwired: 7 in, 1 out]
            }
            n532 = call "FormatStringArray.vi"("strings"=w1220) -> ("value"=w1225:string)  [unwired: 1 in]
            n533 = call "BundleItem.vi"("Value"=w1225, "Key"="pages") -> ("Item"=w1224:T4)
          }
          frame 3 {
            n534 = call "Read Multiple colors.vi"("Tab in"=w1233) -> ("Tab out"=w1230:refnum<class "Tab.lvclass">, "Multiple colors"=w1229:bool)  [unwired: 7 in]
            n535 = case shown="False" w1229 {
              tunnel: w1230 -> [w1240 w1246]
              tunnel: [w1239 w1245] -> w1232
              tunnel: [w1237 w1243] -> w1231
              frame False {
                n536 = call "Read Colors.vi"("Tab in"=w1240) -> ("Tab out"=w1239:refnum<class "Tab.lvclass">, "Colors"=w1238:T13)  [unwired: 7 in]
                n537 = Unbundle By Name(w1238) -> ("Background Color"=w1237:u32)
              }
              frame True {
                n538 = call "Read Pages.vi"("PageSelector in"=w1246) -> ("PageSelector out"=w1245:refnum<class "Tab.lvclass">, "Pages"=w1244:refnum<class "Page.lvclass">[])  [unwired: 7 in]
                n539 = Index Array(array=w1244) -> (element=w1241:refnum<class "Page.lvclass">)  [unwired: 1 in]
                n540 = call "Read Colors.vi"("Page in"=w1241) -> ("Colors"=w1242:T13)  [unwired: 7 in, 1 out]
                n541 = Unbundle By Name(w1242) -> ("Background Color"=w1243:u32)
              }
            }
            n542 = call "FormatColor.vi"("color"=w1231) -> ("value"=w1235:string)
            n543 = call "BundleItem.vi"("Value"=w1235, "Key"="activeBackground") -> ("Item"=w1234:T4)
          }
          frame Default {
          }
        }
      }
    }
    frame "lvSystemTabControl" {
      n544 = call "ToTab.vi"("Generic in"=w1252) -> ("error out"=w1250:errorcluster, "Tab out"=w1251:refnum<class "Tab.lvclass">)  [unwired: 9 in]
      n545 = while {
        shift-right: [w1260] -> w1254
        shift-left: w1251 -> [w1261]
        tunnel: [w1259] -> w1255 mode=indexing
        tunnel: w1253 -> [w1257]
        tunnel: w1250 -> [_]
        tunnel: w1249 -> [w1256]
        i -> [w1262]
        stop <- w1258 stop-if-true
        n546 = case shown="2" w1262 {
          tunnel: w1261 -> [w1263 w1270 w1277 w1284]
          tunnel: [w1263 w1269 w1276 w1284] -> w1260
          tunnel: [w1265 w1271 w1278 _] -> w1259
          tunnel: [_ _ _ TRUE] -> w1258
          tunnel: w1257 -> [w1264 _ _ _]
          tunnel: w1256 -> [_ w1268 _ _]
          frame 0 {
            n547 = call "FormatPoint.vi"("point"=w1264) -> ("value"=w1266:string)
            n548 = call "BundleItem.vi"("Value"=w1266, "Key"="position") -> ("Item"=w1265:T4)
          }
          frame 1 {
            n549 = call-dynamic "GetControlSize.vi"("Control in"=w1270) -> ("Control out"=w1269:refnum<class "Tab.lvclass">)  [unwired: 7 in, 1 out]
            n550 = call "FormatSize.vi"("size"=w1268) -> ("value"=w1272:string)
            n551 = call "BundleItem.vi"("Value"=w1272, "Key"="bounds") -> ("Item"=w1271:T4)
          }
          frame 2 {
            n552 = call "Read Pages.vi"("PageSelector in"=w1277) -> ("PageSelector out"=w1276:refnum<class "Tab.lvclass">, "Pages"=w1275:refnum<class "Page.lvclass">[])  [unwired: 7 in]
            n553 = for {
              tunnel: w1275 -> [w1282] mode=indexing
              tunnel: [w1281] -> w1274 mode=indexing
              n554 = call "Read Label.vi"("Page in"=w1282) -> ("Label"=w1281:string)  [unwired: 7 in, 1 out]
            }
            n555 = call "FormatStringArray.vi"("strings"=w1274) -> ("value"=w1279:string)  [unwired: 1 in]
            n556 = call "BundleItem.vi"("Value"=w1279, "Key"="pages") -> ("Item"=w1278:T4)
          }
          frame Default {
          }
        }
      }
    }
    frame Default {
      n557 = while {
        shift-right: [w1294] -> w1287
        shift-left: w1289 -> [w1295]
        tunnel: [w1293] -> w1288 mode=indexing
        tunnel: w1286 -> [w1291]
        tunnel: w1285 -> [w1290]
        i -> [w1296]
        stop <- w1292 stop-if-true
        n558 = case shown="Default" w1296 {
          tunnel: w1295 -> [w1300 w1303 w1309]
          tunnel: [w1299 w1303 w1309] -> w1294
          tunnel: [w1298 w1305 _] -> w1293
          tunnel: [_ _ TRUE] -> w1292
          tunnel: w1291 -> [_ w1304 _]
          tunnel: w1290 -> [w1297 _ _]
          frame 0 {
            n559 = call "Read Bounds.vi"("GObject in"=w1300) -> ("GObject out"=w1299:refnum<class "Control.lvclass">)  [unwired: 7 in, 1 out]
            n560 = call "FormatSize.vi"("size"=w1297) -> ("value"=w1301:string)
            n561 = call "BundleItem.vi"("Value"=w1301, "Key"="bounds") -> ("Item"=w1298:T4)
          }
          frame 1 {
            n562 = call "FormatPoint.vi"("point"=w1304) -> ("value"=w1306:string)
            n563 = call "BundleItem.vi"("Value"=w1306, "Key"="position") -> ("Item"=w1305:T4)
          }
          frame Default {
          }
        }
      }
    }
  }
  n564 = call "Read PythonConfiguration.vi"("PythonConverter_GUI in"=w6) -> ("PythonConverter_GUI out"=→"PythonConverter_GUI out":refnum<class "PythonConverter_GUI.lvclass">, "PythonConfiguration"=w16:refnum<class "PythonConfiguration.lvclass">)  [unwired: 7 in]
  n565 = call "Read App Configuration Path.vi"("PythonConfiguration in"=w16) -> ("App Configuration Path"=w17:path)  [unwired: 7 in, 1 out]
  n566 = call-dynamic "GetObjectName.vi"("GObject in"=w12) -> ("GObject out"=→"Control out":refnum<class "Control.lvclass">, "Name"=w10:string)  [unwired: 6 in, 1 out]
  n567 = call "WriteItems.vi"("Items"=w14, "section"=w10, "error in"=w5, "Path"=w17) -> ("error out"=→"error out":errorcluster)  [unwired: 5 in]
